vi "NIIE_lv_icon.vi"(10 "Color Icon":T4={"image type"=0, "image depth"=8, "image"=[255, 255, 255, 255, 255, 255, 255, 255, 255, 255, 255, 255, 255, 255, 255, 255, 255, 255, 255, 255, 255, 255, 255, 255, 255, 255, 255, 255, 255, 255, 255, 255, 255, 0, 0, 0, 0, 0, 0, 0, 0, 0, 0, 0, 0, 0, 0, 0, 0, 0, 0, 0, 0, 0, 0, 0, 0, 0, 0, 0, 0, 0, 0, 255, 255, 0, 0, 0, 0, 0, 0, 0, 0, 0, 0, 0, 0, 0, 0, 0, 0, 0, 0, 0, 0, 0, 0, 0, 0, 0, 0, 0, 0, 0, 0, 255, 255, 0, 0, 255, 255, 255, 255, 255, 255, 255, 255, 255, 255, 255, 255, 255, 255, 255, 255, 255, 255, 255, 0, 0, 0, 0, 0, 0, 0, 0, 0, 255, 255, 0, 0, 255, 250, 250, 250, 250, 250, 250, 250, 250, 250, 250, 250, 250, 248, 250, 44, 250, 44, 255, 0, 0, 0, 0, 0, 0, 0, 0, 0, 255, 255, 0, 0, 255, 250, 255, 255, 255, 255, 255, 255, 255, 255, 255, 255, 255, 248, 250, 44, 250, 44, 255, 0, 0, 0, 0, 0, 0, 0, 0, 0, 255, 255, 0, 0, 255, 250, 255, 209, 197, 209, 255, 255, 255, 209, 197, 209, 255, 248, 252, 43, 252, 44, 255, 0, 0, 0, 0, 0, 0, 0, 0, 0, 255, 255, 0, 0, 255, 250, 255, 197, 255, 197, 255, 255, 255, 197, 255, 197, 255, 248, 44, 44, 44, 44, 255, 0, 0, 0, 0, 0, 0, 0, 0, 0, 255, 255, 0, 0, 255, 250, 209, 197, 255, 197, 209, 255, 209, 197, 255, 197, 209, 248, 43, 252, 43, 44, 255, 0, 0, 0, 0, 0, 0, 0, 0, 0, 255, 255, 0, 0, 255, 250, 197, 209, 255, 209, 197, 255, 197, 209, 255, 209, 197, 248, 252, 8, 252, 44, 255, 0, 0, 0, 0, 0, 0, 0, 0, 0, 255, 255, 0, 0, 255, 250, 197, 255, 255, 255, 197, 255, 197, 255, 255, 255, 197, 248, 252, 8, 252, 44, 255, 0, 0, 0, 0, 0, 0, 0, 0, 0, 255, 255, 0, 0, 255, 250, 255, 255, 255, 255, 209, 197, 209, 255, 255, 255, 255, 248, 43, 252, 43, 44, 255, 0, 0, 0, 0, 0, 0, 0, 0, 0, 255, 255, 0, 0, 255, 250, 255, 255, 255, 255, 255, 255, 255, 255, 255, 255, 255, 248, 44, 44, 44, 44, 255, 0, 0, 0, 0, 0, 0, 0, 0, 0, 255, 255, 0, 0, 255, 248, 248, 248, 248, 248, 248, 248, 248, 248, 248, 248, 248, 248, 44, 44, 131, 131, 255, 0, 0, 0, 0, 0, 0, 0, 0, 0, 255, 255, 0, 0, 255, 44, 44, 44, 44, 44, 44, 44, 44, 44, 44, 44, 44, 44, 44, 44, 131, 5, 131, 131, 0, 0, 0, 0, 0, 0, 0, 0, 255, 255, 0, 0, 255, 44, 252, 44, 44, 44, 44, 44, 252, 44, 44, 44, 44, 35, 35, 35, 131, 5, 5, 5, 131, 131, 0, 0, 0, 0, 0, 0, 255, 255, 0, 0, 255, 252, 213, 252, 44, 44, 44, 252, 35, 252, 44, 35, 35, 44, 44, 44, 131, 5, 5, 255, 5, 5, 131, 131, 0, 0, 0, 0, 255, 255, 0, 0, 255, 44, 212, 44, 44, 44, 44, 35, 44, 44, 35, 44, 44, 44, 44, 44, 131, 5, 255, 255, 255, 5, 5, 5, 131, 35, 35, 0, 255, 255, 0, 0, 255, 255, 213, 255, 255, 255, 35, 255, 255, 35, 255, 255, 255, 255, 255, 255, 131, 5, 5, 255, 5, 5, 131, 131, 0, 0, 0, 0, 255, 255, 0, 0, 0, 0, 212, 0, 0, 0, 35, 0, 0, 35, 0, 0, 213, 212, 212, 213, 131, 5, 5, 5, 131, 131, 0, 0, 0, 0, 0, 0, 255, 255, 0, 0, 0, 0, 0, 213, 0, 0, 0, 35, 35, 0, 0, 212, 0, 0, 0, 0, 131, 5, 131, 131, 0, 0, 0, 0, 0, 0, 0, 0, 255, 255, 0, 0, 0, 0, 0, 0, 212, 212, 0, 0, 0, 0, 213, 0, 0, 0, 0, 0, 131, 131, 0, 0, 0, 0, 0, 0, 0, 0, 0, 0, 255, 255, 0, 0, 0, 0, 0, 0, 0, 0, 213, 212, 213, 212, 0, 0, 0, 0, 0, 0, 0, 0, 0, 0, 0, 0, 255, 255, 0, 0, 0, 0, 255, 255, 0, 0, 0, 0, 0, 0, 0, 0, 0, 0, 0, 0, 0, 0, 0, 0, 0, 0, 0, 0, 0, 0, 0, 255, 0, 0, 255, 0, 0, 0, 255, 255, 0, 0, 0, 0, 0, 0, 0, 0, 0, 0, 0, 0, 0, 0, 0, 0, 0, 0, 0, 0, 0, 0, 0, 0, 0, 0, 255, 0, 0, 0, 255, 255, 0, 0, 0, 0, 0, 0, 0, 0, 0, 0, 0, 0, 0, 0, 0, 0, 0, 0, 0, 0, 0, 0, 0, 0, 255, 255, 0, 0, 0, 0, 255, 255, 0, 0, 0, 0, 0, 0, 0, 0, 0, 0, 0, 0, 0, 0, 0, 0, 0, 0, 0, 0, 0, 0, 0, 0, 0, 0, 255, 0, 0, 0, 255, 255, 0, 0, 0, 0, 0, 0, 0, 0, 0, 0, 0, 0, 0, 0, 0, 0, 0, 0, 0, 0, 0, 0, 0, 255, 0, 0, 255, 0, 0, 0, 255, 255, 0, 0, 0, 0, 0, 0, 0, 0, 0, 0, 0, 0, 0, 0, 0, 0, 0, 0, 0, 0, 0, 0, 0, 0, 255, 255, 0, 0, 0, 0, 255, 255, 0, 0, 0, 0, 0, 0, 0, 0, 0, 0, 0, 0, 0, 0, 0, 0, 0, 0, 0, 0, 0, 0, 0, 0, 0, 0, 0, 0, 0, 0, 255, 255, 0, 0, 0, 0, 0, 0, 0, 0, 0, 0, 0, 0, 0, 0, 0, 0, 0, 0, 0, 0, 0, 0, 0, 0, 0, 0, 0, 0, 0, 0, 255, 255, 255, 255, 255, 255, 255, 255, 255, 255, 255, 255, 255, 255, 255, 255, 255, 255, 255, 255, 255, 255, 255, 255, 255, 255, 255, 255, 255, 255, 255, 255, 255], "mask"=[], "colors"=[16777215, 16777164, 16777113, 16777062, 16777011, 16776960, 16764159, 16764108, 16764057, 16764006, 16763955, 16763904, 16751103, 16751052, 16751001, 16750950, 16750899, 16750848, 16738047, 16737996, 16737945, 16737894, 16737843, 16737792, 16724991, 16724940, 16724889, 16724838, 16724787, 16724736, 16711935, 16711884, 16711833, 16711782, 16711731, 16711680, 13434879, 13434828, 13434777, 13434726, 13434675, 13434624, 13421823, 13421772, 13421721, 13421670, 13421619, 13421568, 13408767, 13408716, 13408665, 13408614, 13408563, 13408512, 13395711, 13395660, 13395609, 13395558, 13395507, 13395456, 13382655, 13382604, 13382553, 13382502, 13382451, 13382400, 13369599, 13369548, 13369497, 13369446, 13369395, 13369344, 10092543, 10092492, 10092441, 10092390, 10092339, 10092288, 10079487, 10079436, 10079385, 10079334, 10079283, 10079232, 10066431, 10066380, 10066329, 10066278, 10066227, 10066176, 10053375, 10053324, 10053273, 10053222, 10053171, 10053120, 10040319, 10040268, 10040217, 10040166, 10040115, 10040064, 10027263, 10027212, 10027161, 10027110, 10027059, 10027008, 6750207, 6750156, 6750105, 6750054, 6750003, 6749952, 6737151, 6737100, 6737049, 6736998, 6736947, 6736896, 6724095, 6724044, 6723993, 6723942, 6723891, 6723840, 6711039, 6710988, 6710937, 6710886, 6710835, 6710784, 6697983, 6697932, 6697881, 6697830, 6697779, 6697728, 6684927, 6684876, 6684825, 6684774, 6684723, 6684672, 3407871, 3407820, 3407769, 3407718, 3407667, 3407616, 3394815, 3394764, 3394713, 3394662, 3394611, 3394560, 3381759, 3381708, 3381657, 3381606, 3381555, 3381504, 3368703, 3368652, 3368601, 3368550, 3368499, 3368448, 3355647, 3355596, 3355545, 3355494, 3355443, 3355392, 3342591, 3342540, 3342489, 3342438, 3342387, 3342336, 65535, 65484, 65433, 65382, 65331, 65280, 52479, 52428, 52377, 52326, 52275, 52224, 39423, 39372, 39321, 39270, 39219, 39168, 26367, 26316, 26265, 26214, 26163, 26112, 13311, 13260, 13209, 13158, 13107, 13056, 255, 204, 153, 102, 51, 15597568, 14483456, 12255232, 11141120, 8912896, 7798784, 5570560, 4456448, 2228224, 1114112, 60928, 56576, 47872, 43520, 34816, 30464, 21760, 17408, 8704, 4352, 238, 221, 187, 170, 136, 119, 85, 68, 34, 17, 15658734, 14540253, 12303291, 11184810, 8947848, 7829367, 5592405, 4473924, 2236962, 1118481, 0], "Rectangle"={"left"=0, "top"=0, "right"=32, "bottom"=32}}, 11 "BW Icon":T4={"image type"=0, "image depth"=1, "image"=[255, 255, 255, 255, 128, 0, 0, 1, 128, 0, 0, 1, 159, 255, 252, 1, 144, 0, 84, 1, 151, 255, 84, 1, 150, 251, 84, 1, 149, 117, 4, 1, 149, 117, 36, 1, 147, 174, 84, 1, 147, 174, 84, 1, 151, 223, 36, 1, 151, 255, 4, 1, 144, 0, 28, 1, 144, 0, 22, 1, 148, 16, 241, 129, 158, 59, 18, 97, 148, 36, 23, 29, 159, 255, 242, 97, 132, 73, 241, 129, 130, 50, 22, 1, 129, 132, 24, 1, 128, 120, 0, 97, 128, 0, 0, 145, 128, 0, 0, 17, 128, 0, 0, 97, 128, 0, 0, 17, 128, 0, 0, 145, 128, 0, 0, 97, 128, 0, 0, 1, 128, 0, 0, 1, 255, 255, 255, 255], "mask"=[], "colors"=[16777215, 0], "Rectangle"={"left"=0, "top"=0, "right"=32, "bottom"=32}}) -> (0 "Error Code Out":i32=43, 2 "Color Icon Out":T4={"image type"=0, "image depth"=24, "image"=array[3072 elements], "mask"=[0, 0, 0, 0, 0, 0, 0, 0, 0, 0, 0, 0, 0, 0, 0, 0, 0, 0, 0, 0, 0, 0, 0, 0, 0, 0, 0, 0, 0, 0, 0, 0, 0, 0, 0, 0, 0, 0, 0, 0, 0, 0, 0, 0, 0, 0, 0, 0, 0, 0, 0, 0, 0, 0, 0, 0, 0, 0, 0, 0, 0, 0, 0, 0, 0, 0, 0, 0, 0, 0, 0, 0, 0, 0, 0, 0, 0, 0, 0, 0, 0, 0, 0, 0, 0, 0, 0, 0, 0, 0, 0, 0, 0, 0, 0, 0, 0, 0, 0, 0, 0, 0, 0, 0, 0, 0, 0, 0, 0, 0, 0, 0, 0, 0, 0, 0, 0, 0, 0, 0, 0, 0, 0, 0, 0, 0, 0, 0], "colors"=[], "Rectangle"={"left"=0, "top"=0, "right"=32, "bottom"=32}}, 3 "BW Icon Out":T4={"image type"=0, "image depth"=1, "image"=[0, 0, 0, 0, 0, 0, 0, 0, 0, 0, 0, 0, 0, 0, 0, 0, 0, 0, 0, 0, 0, 0, 0, 0, 0, 0, 0, 0, 0, 0, 0, 0, 0, 0, 0, 0, 0, 0, 0, 0, 0, 0, 0, 0, 0, 0, 0, 0, 0, 0, 0, 0, 0, 0, 0, 0, 0, 0, 0, 0, 0, 0, 0, 0, 0, 0, 0, 0, 0, 0, 0, 0, 0, 0, 0, 0, 0, 0, 0, 0, 0, 0, 0, 0, 0, 0, 0, 0, 0, 0, 0, 0, 0, 0, 0, 0, 0, 0, 0, 0, 0, 0, 0, 0, 0, 0, 0, 0, 0, 0, 0, 0, 0, 0, 0, 0, 0, 0, 0, 0, 0, 0, 0, 0, 0, 0, 0, 0], "mask"=[], "colors"=[16777215, 0], "Rectangle"={"left"=0, "top"=0, "right"=32, "bottom"=32}})   [LabVIEW 2021, in "lv_icon.lvlib"]
doc: "<p>Display this dialog box in one of the following ways:</p>\n\n<ul>\n<li>Double-click the <a href=\"nihelplauncher://docs/csh?context=lvcore_lvconcepts_using_icons\">icon</a> in the upper right corner of the front panel window, block diagram window, or <a href=\"nihelplauncher://docs/csh?context=lvcore_lvconcepts_custom_cont_ind_type\">Control Editor</a> window.</li>\n<li>Right-click the icon in the upper right corner of the front panel window, block diagram window, or <strong>Control Editor</strong> window and select <strong>Edit Icon</strong> from the shortcut menu.</li>\n<li>Select <strong>File<span class=\"U+187\">>></span>VI Properties</strong> or <strong>File<span class=\"U+187\">>></span>Control Properties</strong> to display the <a href=\"nihelplauncher://docs/csh?context=lvcore_lvdialog_vi_properties_dialog_box\">VI Properties</a> dialog box or <strong>Control Properties</strong> dialog box, respectively. Then select <strong>General</strong> from the <strong>Category</strong> pull-down menu and click the <strong>Edit Icon</strong> button.</li>\n<li>Right-click a project library, statechart, class, or XControl item in the <a href=\"nihelplauncher://docs/csh?context=lvcore_lvconcepts_using_labview_projects\">Project Explorer</a> window and select <strong> Properties</strong> from the shortcut menu to display the corresponding <strong>Properties</strong> dialog box. Then click the <strong>Edit</strong> button on the <strong>General Settings</strong> page.</li>\n</ul>\n\n<p>Use this dialog box to <a href=\"nihelplauncher://docs/csh?context=lvcore_lvhowto_creating_icons\">create and edit icons</a>.</p>"
uses:
  vi.lib/LabVIEW Icon API/lv_icon/lv_icon.lvlib
  MB CORE/TypeDefs/Cluster_BodyText.ctl
  vi.lib/LabVIEW Icon API/lv_icon/Controls/Font.ctl
  vi.lib/LabVIEW Icon API/lv_icon/Controls/Alignment.ctl
  MB CORE/TypeDefs/Cluster_Layer Data.ctl
  NIIconEditor/Controls/LayerList.ctl
  NIIconEditor/Controls/NewLayer.ctl
  NIIconEditor/Controls/DeleteLayer.ctl
  NIIconEditor/Controls/Arrow Up.ctl
  NIIconEditor/Controls/Arrow Down.ctl
  NIIconEditor/Controls/Framework Templates.ctl
  vi.lib/LabVIEW Icon API/lv_icon/Controls/Graphic.ctl
  NIIconEditor/Controls/ColorChange.ctl
  vi.lib/LabVIEW Icon API/lv_icon/Controls/IEColor.ctl
  NIIconEditor/Controls/Rotate.ctl
  NIIconEditor/Controls/Flip.ctl
  MB CORE/TypeDefs/Cluster_Button Draw Tools.ctl
  MB CORE/TypeDefs/Bool_Draw Tool.ctl
  MB CORE/TypeDefs/Bool_Line Tool.ctl
  MB CORE/TypeDefs/Bool_ColorExtractor Tool.ctl
  MB CORE/TypeDefs/Bool_Fill Tool.ctl
  MB CORE/TypeDefs/Bool_IERect Tool.ctl
  MB CORE/TypeDefs/Bool_FRect Tool.ctl
  MB CORE/TypeDefs/Bool_Circle Tool.ctl
  MB CORE/TypeDefs/Bool_FillCircle Tool.ctl
  MB CORE/TypeDefs/Bool_Eraser Tool.ctl
  MB CORE/TypeDefs/Bool_Text Tool.ctl
  MB CORE/TypeDefs/Bool_Selection Tool.ctl
  MB CORE/TypeDefs/Bool_Move Tool.ctl
  MB CORE/TypeDefs/String_TextMarker Tool.ctl
  <vilib>/picture/picture.llb/imagedata.ctl
  MB CORE/TypeDefs/Cluster_Path&Icon.ctl
  NIIconEditor/Controls/Refresh.ctl
  <vilib>/Utility/miscctls.llb/LVKeyNavTypeDef.ctl
  NIIconEditor/Controls/References Cluster.ctl
  <vilib>/Utility/miscctls.llb/LVPoint32TypeDef.ctl
  <vilib>/Utility/miscctls.llb/LVPositionTypeDef.ctl
  vi.lib/LabVIEW Icon API/lv_icon/Controls/Pathes.ctl
  NIIconEditor/Class/Ants/Ants.lvclass
  NIIconEditor/Class/FakedArray/FakedArray.lvclass
  vi.lib/LabVIEW Icon API/lv_icon/Classes/Icon/Icon.lvclass
  NIIconEditor/Class/Icon Library/Glyph.lvclass
  <resource>/dialog/lvconfig.llb/LV Config Read String.vi
  <resource>/dialog/lvconfig.llb/LV Config Write String.vi
panel:
  out "LabVIEW Icon out":string
  in  "LabVIEW Icon in":string
  out "Terminals":picture
  out "Preview2":picture
  in  "?":cluster{T1[], i32, bool}
  out "TextMarker":T2="^"
  in  "Help":bool
  in  "Cancel":bool
  in  "OK":bool
  out "XYZ":string="X: 14\nY: 31\nZ: 1"
  out "RGB":string="R: 0\nG: 0\nB: 0"
  out "Icon":picture
  out "Clipboard":picture
  in  "?":T3[](array[typedef])
  in  "Tab Control":T5(tab)
  in  "refreshTemplates":T6
  out "templates path str":string
  in  "Templates":string(tree)="<All>"
  in  "Filter templates by keyword":string
  in  "Framework Templates":T7={"Scrollbar"=0, "Path & Icon 1"={"Rectangle"={"left"=0, "top"=0, "right"=32, "bottom"=32}, "Path"=path "C:/Users/tsandris/Documents/LabVIEW Data/Icon Templates/VI/Frameworks/_blank.png", "Image"=bytes[3230], "Filter"="VI\\Frameworks", "FileName"="_blank"}, "Path & Icon 2"={"Rectangle"={"left"=0, "top"=0, "right"=32, "bottom"=32}, "Path"=path "C:/Users/tsandris/Documents/LabVIEW Data/Icon Templates/Library/Frameworks/_blank.png", "Image"=bytes[3230], "Filter"="Library\\Frameworks", "FileName"="_blank"}, "Path & Icon 3"={"Rectangle"={"left"=0, "top"=0, "right"=0, "bottom"=0}, "Path"=path "", "Image"=bytes[0], "Filter"="", "FileName"=""}, "Path & Icon 4"={"Rectangle"={"left"=0, "top"=0, "right"=0, "bottom"=0}, "Path"=path "", "Image"=bytes[0], "Filter"="", "FileName"=""}, "Path & Icon 5"={"Rectangle"={"left"=0, "top"=0, "right"=0, "bottom"=0}, "Path"=path "", "Image"=bytes[0], "Filter"="", "FileName"=""}, "Path & Icon 6"={"Rectangle"={"left"=0, "top"=0, "right"=0, "bottom"=0}, "Path"=path "", "Image"=bytes[0], "Filter"="", "FileName"=""}, "Path & Icon 7"={"Rectangle"={"left"=0, "top"=0, "right"=0, "bottom"=0}, "Path"=path "", "Image"=bytes[0], "Filter"="", "FileName"=""}, "Path & Icon 8"={"Rectangle"={"left"=0, "top"=0, "right"=0, "bottom"=0}, "Path"=path "", "Image"=bytes[0], "Filter"="", "FileName"=""}, "Path & Icon 9"={"Rectangle"={"left"=0, "top"=0, "right"=0, "bottom"=0}, "Path"=path "", "Image"=bytes[0], "Filter"="", "FileName"=""}, "Path & Icon 10"={"Rectangle"={"left"=0, "top"=0, "right"=0, "bottom"=0}, "Path"=path "", "Image"=bytes[0], "Filter"="", "FileName"=""}, "Path & Icon 11"={"Rectangle"={"left"=0, "top"=0, "right"=0, "bottom"=0}, "Path"=path "", "Image"=bytes[0], "Filter"="", "FileName"=""}, "Path & Icon 12"={"Rectangle"={"left"=0, "top"=0, "right"=0, "bottom"=0}, "Path"=path "", "Image"=bytes[0], "Filter"="", "FileName"=""}, "Path & Icon 13"={"Rectangle"={"left"=0, "top"=0, "right"=0, "bottom"=0}, "Path"=path "", "Image"=bytes[0], "Filter"="", "FileName"=""}, "Path & Icon 14"={"Rectangle"={"left"=0, "top"=0, "right"=0, "bottom"=0}, "Path"=path "", "Image"=bytes[0], "Filter"="", "FileName"=""}, "Path & Icon 15"={"Rectangle"={"left"=0, "top"=0, "right"=0, "bottom"=0}, "Path"=path "", "Image"=bytes[0], "Filter"="", "FileName"=""}, "Path & Icon 16"={"Rectangle"={"left"=0, "top"=0, "right"=0, "bottom"=0}, "Path"=path "", "Image"=bytes[0], "Filter"="", "FileName"=""}, "Path & Icon 17"={"Rectangle"={"left"=0, "top"=0, "right"=0, "bottom"=0}, "Path"=path "", "Image"=bytes[0], "Filter"="", "FileName"=""}, "Path & Icon 18"={"Rectangle"={"left"=0, "top"=0, "right"=0, "bottom"=0}, "Path"=path "", "Image"=bytes[0], "Filter"="", "FileName"=""}, "Path & Icon 19"={"Rectangle"={"left"=0, "top"=0, "right"=0, "bottom"=0}, "Path"=path "", "Image"=bytes[0], "Filter"="", "FileName"=""}, "Path & Icon 20"={"Rectangle"={"left"=0, "top"=0, "right"=0, "bottom"=0}, "Path"=path "", "Image"=bytes[0], "Filter"="", "FileName"=""}, "Path & Icon 21"={"Rectangle"={"left"=0, "top"=0, "right"=0, "bottom"=0}, "Path"=path "", "Image"=bytes[0], "Filter"="", "FileName"=""}, "Path & Icon 22"={"Rectangle"={"left"=0, "top"=0, "right"=0, "bottom"=0}, "Path"=path "", "Image"=bytes[0], "Filter"="", "FileName"=""}, "Path & Icon 23"={"Rectangle"={"left"=0, "top"=0, "right"=0, "bottom"=0}, "Path"=path "", "Image"=bytes[0], "Filter"="", "FileName"=""}, "Path & Icon 24"={"Rectangle"={"left"=0, "top"=0, "right"=0, "bottom"=0}, "Path"=path "", "Image"=bytes[0], "Filter"="", "FileName"=""}, "Path & Icon 25"={"Rectangle"={"left"=0, "top"=0, "right"=0, "bottom"=0}, "Path"=path "", "Image"=bytes[0], "Filter"="", "FileName"=""}, "Path & Icon 26"={"Rectangle"={"left"=0, "top"=0, "right"=0, "bottom"=0}, "Path"=path "", "Image"=bytes[0], "Filter"="", "FileName"=""}, "Path & Icon 27"={"Rectangle"={"left"=0, "top"=0, "right"=0, "bottom"=0}, "Path"=path "", "Image"=bytes[0], "Filter"="", "FileName"=""}, "Path & Icon 28"={"Rectangle"={"left"=0, "top"=0, "right"=0, "bottom"=0}, "Path"=path "", "Image"=bytes[0], "Filter"="", "FileName"=""}, "Path & Icon 29"={"Rectangle"={"left"=0, "top"=0, "right"=0, "bottom"=0}, "Path"=path "", "Image"=bytes[0], "Filter"="", "FileName"=""}, "Path & Icon 30"={"Rectangle"={"left"=0, "top"=0, "right"=0, "bottom"=0}, "Path"=path "", "Image"=bytes[0], "Filter"="", "FileName"=""}}
  in  "Body Text":T8={"Line 1 text"="", "Line 2 text"="", "Line 3 text"="", "Line 4 text"="", "Line 1 color"=0, "Line 2 color"=0, "Line 3 color"=0, "Line 4 color"=0, "Body Text Spec"={"Font"="", "Alignment"=1, "Size"=9}, "Center text vertically"=TRUE, "Capitalize Text"=TRUE} {"Body Text Spec"."Alignment" items=["left", "center", "right"]}
  in  "Filter glyphs by keyword":string
  in  "Glyphs":string(tree)="<All>"
  out "glyph path str":string
  out "Glyphs []":T1[][](array[typedef])
  in  "refreshGlyphs":T6
  in  "Add Layer":T11
  in  "Remove Layer":T12
  in  "Move Down":T13
  in  "Move Up":T14
  in  "Icon Template":T15={"LayerIcon"=bytes[0], "LayerName"="", "Opacity"=100, "Visibility?"=TRUE} {"Opacity" scale=0.0..100.0}
  in  "Icon Text":T15={"LayerIcon"=bytes[0], "LayerName"="Icon Text", "Opacity"=100, "Visibility?"=TRUE} {"Opacity" scale=0.0..100.0}
  in  "User Layers":T16={"Scrollbar"=0, "Layer 1"={"LayerIcon"=bytes[3230], "LayerName"="VI Icon", "Opacity"=100, "Visibility?"=TRUE}, "Layer 2"={"LayerIcon"=bytes[3230], "LayerName"="", "Opacity"=100, "Visibility?"=TRUE}, "Layer 3"={"LayerIcon"=bytes[3230], "LayerName"="", "Opacity"=100, "Visibility?"=TRUE}, "Layer 4"={"LayerIcon"=bytes[3230], "LayerName"="", "Opacity"=100, "Visibility?"=TRUE}} {"Layer 4"."Opacity" scale=0.0..100.0; "Layer 3"."Opacity" scale=0.0..100.0; "Layer 2"."Opacity" scale=0.0..100.0; "Layer 1"."Opacity" scale=0.0..100.0}
  out "Preview":picture
  in  "Horizontal Flip":T17
  in  "Clockwise Rotate":T18
  in  "Swap":T19
  in  "Line Color":T20
  in  "Fill Color":T20=16777215
  in  "Tools":T21=enum."Rectangle"
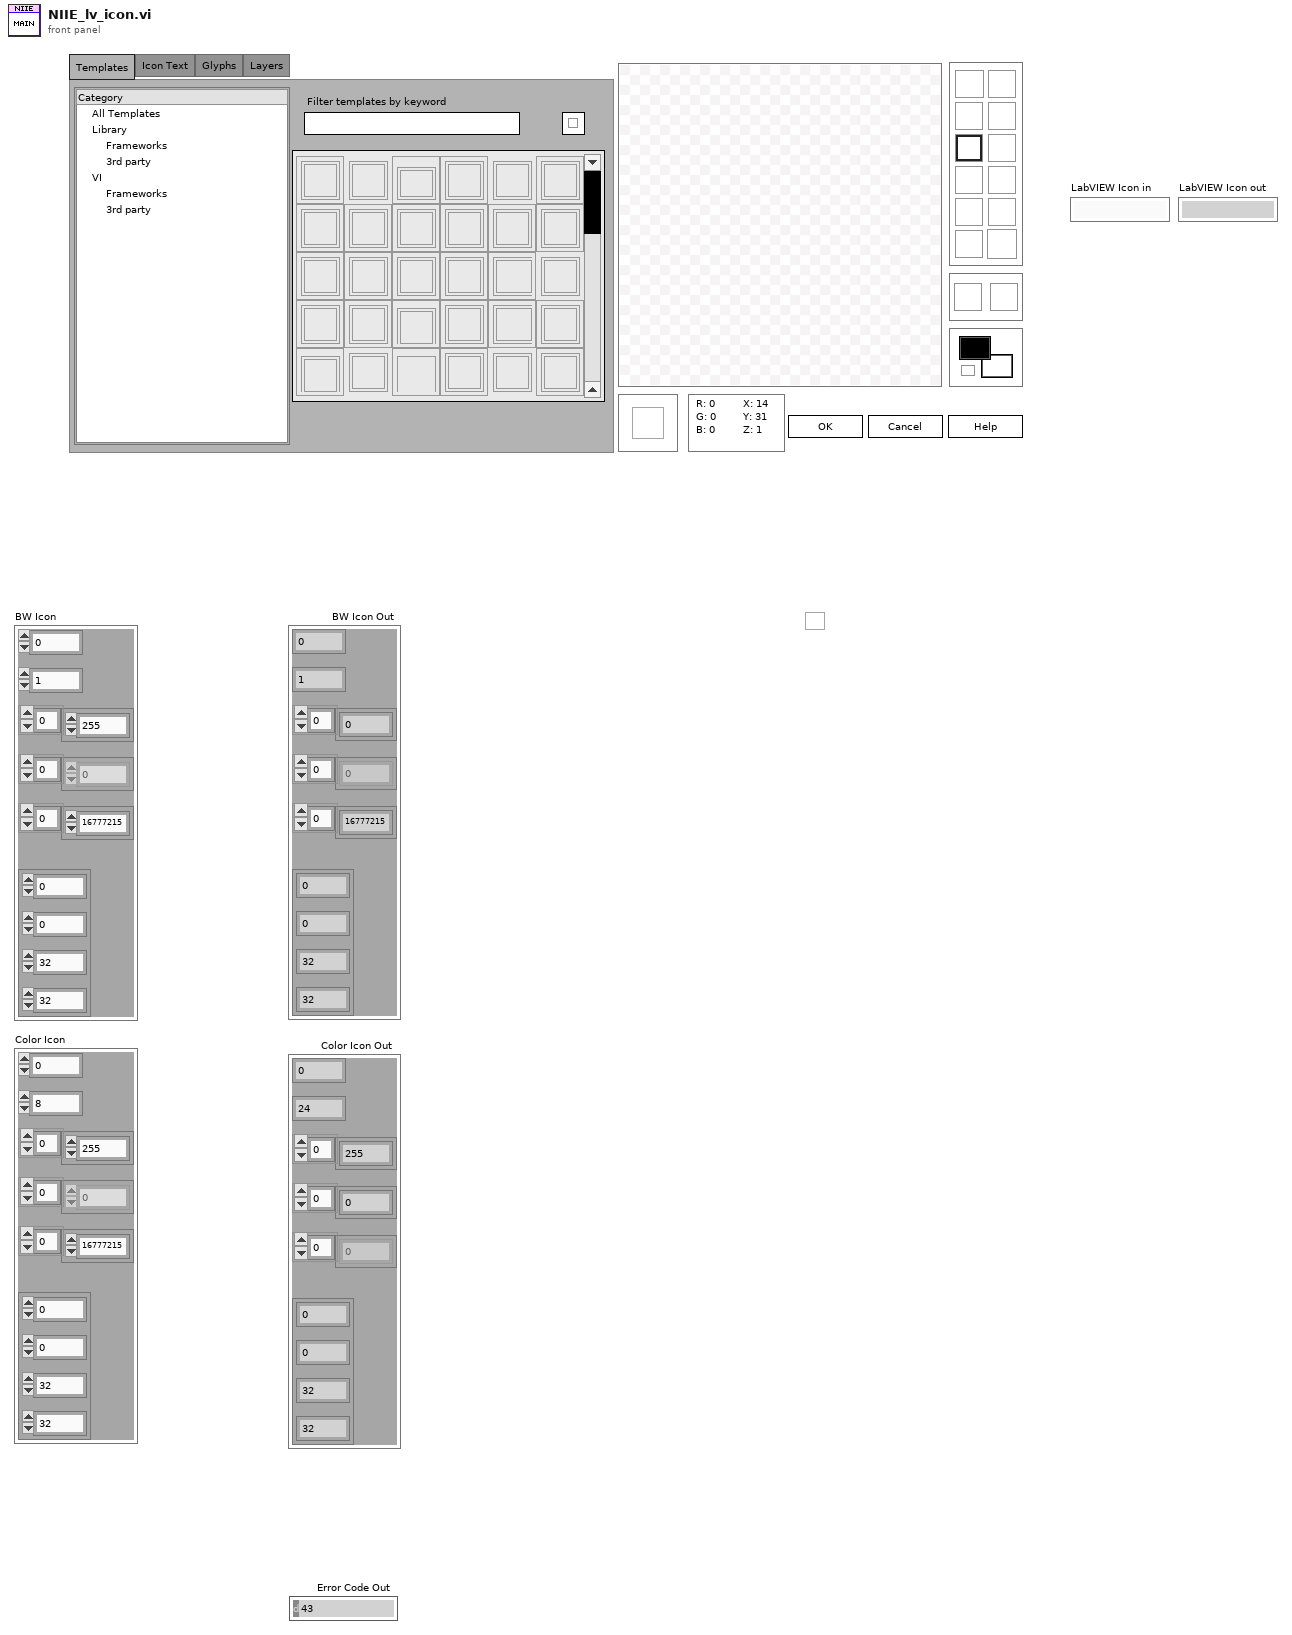
[diagram p1: front panel]
types:
  T1 = typedef "Graphic.ctl" = cluster{"Rectangle":cluster{"left":i16, "top":i16, "right":i16, "bottom":i16}, "Path":path, "Image":picture, "Filter":string, "FileName":string}
  T2 = typedef "String_TextMarker Tool.ctl" = string
  T3 = typedef "Cluster_Path&Icon.ctl" = cluster{"Rectangle":cluster{"left":i16, "top":i16, "right":i16, "bottom":i16}, "Path":path, "Image":picture, "Filter":string, "FileName":string}
  T4 = typedef "imagedata.ctl" = cluster{"image type":i32, "image depth":i32, "image":u8[], "mask":u8[], "colors":u32[], "Rectangle":cluster{"left":i16, "top":i16, "right":i16, "bottom":i16}}
  T5 = enum32{"Templates", "Icon Text", "Glyphs", "Layers"}
  T6 = typedef "Refresh.ctl" = bool
  T7 = typedef "Framework Templates.ctl" = cluster{"Scrollbar":i32, "Path & Icon 1":T1, "Path & Icon 2":T1, "Path & Icon 3":T1, "Path & Icon 4":T1, "Path & Icon 5":T1, "Path & Icon 6":T1, "Path & Icon 7":T1, "Path & Icon 8":T1, "Path & Icon 9":T1, "Path & Icon 10":T1, "Path & Icon 11":T1, "Path & Icon 12":T1, "Path & Icon 13":T1, "Path & Icon 14":T1, "Path & Icon 15":T1, "Path & Icon 16":T1, "Path & Icon 17":T1, "Path & Icon 18":T1, "Path & Icon 19":T1, "Path & Icon 20":T1, "Path & Icon 21":T1, "Path & Icon 22":T1, "Path & Icon 23":T1, "Path & Icon 24":T1, "Path & Icon 25":T1, "Path & Icon 26":T1, "Path & Icon 27":T1, "Path & Icon 28":T1, "Path & Icon 29":T1, "Path & Icon 30":T1}
  T8 = typedef "Cluster_BodyText.ctl" = cluster{"Line 1 text":string, "Line 2 text":string, "Line 3 text":string, "Line 4 text":string, "Line 1 color":u32, "Line 2 color":u32, "Line 3 color":u32, "Line 4 color":u32, "Body Text Spec":cluster{"Font":T9, "Alignment":T10, "Size":u8}, "Center text vertically":bool, "Capitalize Text":bool}
  T9 = typedef "Font.ctl" = string
  T10 = typedef "Alignment.ctl" = u16
  T11 = typedef "NewLayer.ctl" = bool
  T12 = typedef "DeleteLayer.ctl" = bool
  T13 = typedef "Arrow Down.ctl" = bool
  T14 = typedef "Arrow Up.ctl" = bool
  T15 = typedef "Cluster_Layer Data.ctl" = cluster{"LayerIcon":picture, "LayerName":string, "Opacity":u8, "Visibility?":bool}
  T16 = typedef "LayerList.ctl" = cluster{"Scrollbar":i32, "Layer 1":T15, "Layer 2":T15, "Layer 3":T15, "Layer 4":T15}
  T17 = typedef "Flip.ctl" = bool
  T18 = typedef "Rotate.ctl" = bool
  T19 = typedef "ColorChange.ctl" = bool
  T20 = typedef "IEColor.ctl" = u32
  T21 = typedef "Cluster_Button Draw Tools.ctl" = enum32{"Pencil", "Line", "Dropper", "Fill", "Rectangle", "Filled Rectangle", "Ellipse", "Filled Ellipse", "Eraser", "Text", "Select", "Move"}
  T22 = enum32{"Invalid", "Standard", "Closed", "Hidden", "Minimized", "Maximized"}
  T23 = typedef "References Cluster.ctl" = cluster{"Add Layer":refnum<vi>, "Remove Layer":refnum<vi>, "Line Text":refnum<vi>[], "Body Text Spec":refnum<vi>, "DNL_Font":refnum<vi>, "glyph path str":refnum<vi>, "templates path str":refnum<vi>, "Arrow Up":refnum<vi>, "Arrow Down":refnum<vi>, "IE VI Ref":refnum<vi>, "Glyphs tree":refnum<vi>, "Templates tree":refnum<vi>, "Layer Icon Text":refnum<vi>, "Layer Template":refnum<vi>, "Clipboard":refnum<vi>, "BW icon in":refnum<vi>, "Color icon in":refnum<vi>, "Layer Clust":refnum<vi>, "Body Text":refnum<vi>, "DNL_Framework Templates":refnum<vi>, "Search Templates":refnum<vi>, "TextMarker":refnum<vi>, "Tab Control":refnum<vi>, "Search Glyphs":refnum<vi>, "Line Color":refnum<vi>, "DNL_Glyphs []":refnum<vi>, "Fill Color":refnum<vi>, "Tools":refnum<vi>, "Glyphs tree":refnum<vi>, "Icon":refnum<vi>, "Preview":refnum<vi>, "Ants":refnum<vi>, "Terminals":refnum<vi>, "menu reference":refnum<k9>, "LayerNames":refnum<vi>[], "GlyphLoadAnimation":refnum<vi>, "TemplateLoadAnimation":refnum<vi>, "refreshGlyphs":refnum<vi>, "refreshTemplates":refnum<vi>}
  T24 = typedef "LVKeyNavTypeDef.ctl" = cluster{"Control":bool, "Shift":bool, "Key":string}
  T25 = cluster{"Left":i16, "Top":i16, "Right":i16, "Bottom":i16}
  T26 = typedef "LVAllMonitorsDisplayTypeDef.ctl" = cluster{"Bounds":cluster{"Left":i16, "Top":i16, "Right":i16, "Bottom":i16}, "Depth":i16}[]
  T27 = cluster{"Global stop?":refnum<user-event>, "Templates":refnum<user-event>, "Glyphs":refnum<user-event>}
  T28 = typedef "IE Data.ctl" = cluster{"Class":T29, "Ref":T23, "Support":T30}
  T29 = typedef "IE Classes.ctl" = cluster{"Ants":refnum<class "Ants.lvclass">, "Layer":refnum<class "FakedArray.lvclass">, "Templates":refnum<class "FakedArray.lvclass">, "Icon":refnum<class "Icon.lvclass">, "Glyph":refnum<class "Glyph.lvclass">, "Settings":refnum<class "Settings.lvclass">, "Tools":refnum<class "Tools Paint.lvclass">}
  T30 = typedef "SupportClass.ctl" = cluster{"AntsRect":cluster{"left":i16, "top":i16, "right":i16, "bottom":i16}, "Mouse Move Coords":T31, "Mouse Down Coords":T31, "Temp Coord":T31, "Action":T32, "Edge Color":T20, "Fill Color":T20, "Mouse Down?":bool, "Draft Mode?":bool, "Temp Icon":picture, "CTRL Pressed":bool, "Move Selection?":bool, "AntsRect Orig":cluster{"left":i16, "top":i16, "right":i16, "bottom":i16}, "Text":string, "TM Set?":bool, "Mouse inside icon?":bool, "Tool (old value)":u32, "Pencil Move Color":u32, "Swap Colors?":bool, "Shift pressed?":bool}
  T31 = typedef "LVPoint32TypeDef.ctl" = cluster{"Horizontal":i32, "Vertical":i32}
  T32 = typedef "ENUM_SupportClass_Action.ctl" = enum16{"Default", "Move Selection", "Glyph Library", "Tool"}
  T33 = typedef "LVPositionTypeDef.ctl" = cluster{"Left":i32, "Top":i32}
  T34 = typedef "Pathes.ctl" = enum16{"Root Path", "Icon Templates", "Icon Templates VI", "Icon Templates Lib", "Glyphs"}
  T35 = typedef "lveventtype.ctl" = enum32{"Null", "Timeout", "Annotation Menu Selection", "Annotation Menu Selection?", "App Instance Close", "App Instance Close?", "Autoscale Range Change", "Bookmark Info Change", "Cell Edit", "Cell Edit?", "Cursor Grab", "Cursor Grab?", "Cursor Menu Selection", "Cursor Menu Selection?", "Cursor Move", "Cursor Release", "Data Change", "Direction Change", "Display State Change", "Drag Ended", "Drag Enter", "Drag Leave", "Drag Over", "Drag Source Update", "Drag Starting", "Drag Starting?", "Drop", "Exec State Change", "Key Down", "Key Down?", "Key Repeat", "Key Repeat?", "Key Up", "Listbox Double Click", "Menu Activation?", "Menu Selection (App)", "Menu Selection? (App)", "Menu Selection (User)", "Mouse Down", "Mouse Down?", "Mouse Enter", "Mouse Leave", "Mouse Move", "Mouse Up", "Mouse Wheel", "NI Security User Change (App)", "Pane Size", "Panel Close", "Panel Close?", "Panel Resize", "Plot Attribute Change", "Scale Range Change", "Shortcut Menu Activation?", "Shortcut Menu Selection (App)", "Shortcut Menu Selection? (App)", "Shortcut Menu Selection (User)", "Tree Double Click", "Tree Drag", "Tree Drag?", "Tree Drop", "Tree Drop?", "Tree Item Close", "Tree Item Close?", "Tree Item Open", "Tree Item Open?", "User Event", "Value Change"}
  T36 = typedef "eventvkey.ctl" = enum16{"ASCII", "Enter", "Return", "Shift", "Ctrl", "Alt", "Cmd", "Opt", "Caps", "NumLock", "Clear", "Break", "Up", "Down", "Left", "Right", "Insert", "Delete", "Home", "End", "PageUp", "PageDown", "Escape", "Help", "Pause", "ScrollLock", "F1", "F2", "F3", "F4", "F5", "F6", "F7", "F8", "F9", "F10", "F11", "F12", "F13", "F14", "F15", "F16", "F17", "F18", "F19", "F20", "F21", "F22", "F23", "F24", "Play", "VolumeUp", "VolumeDown", "Mute", "Two Byte Char"}
  T37 = cluster{"Shift":bool, "Ctrl":bool, "Alt":bool, "Cmd":bool, "Opt":bool}
  T38 = typedef "LVRectTypeDef.ctl" = cluster{"Left":i16, "Top":i16, "Right":i16, "Bottom":i16}
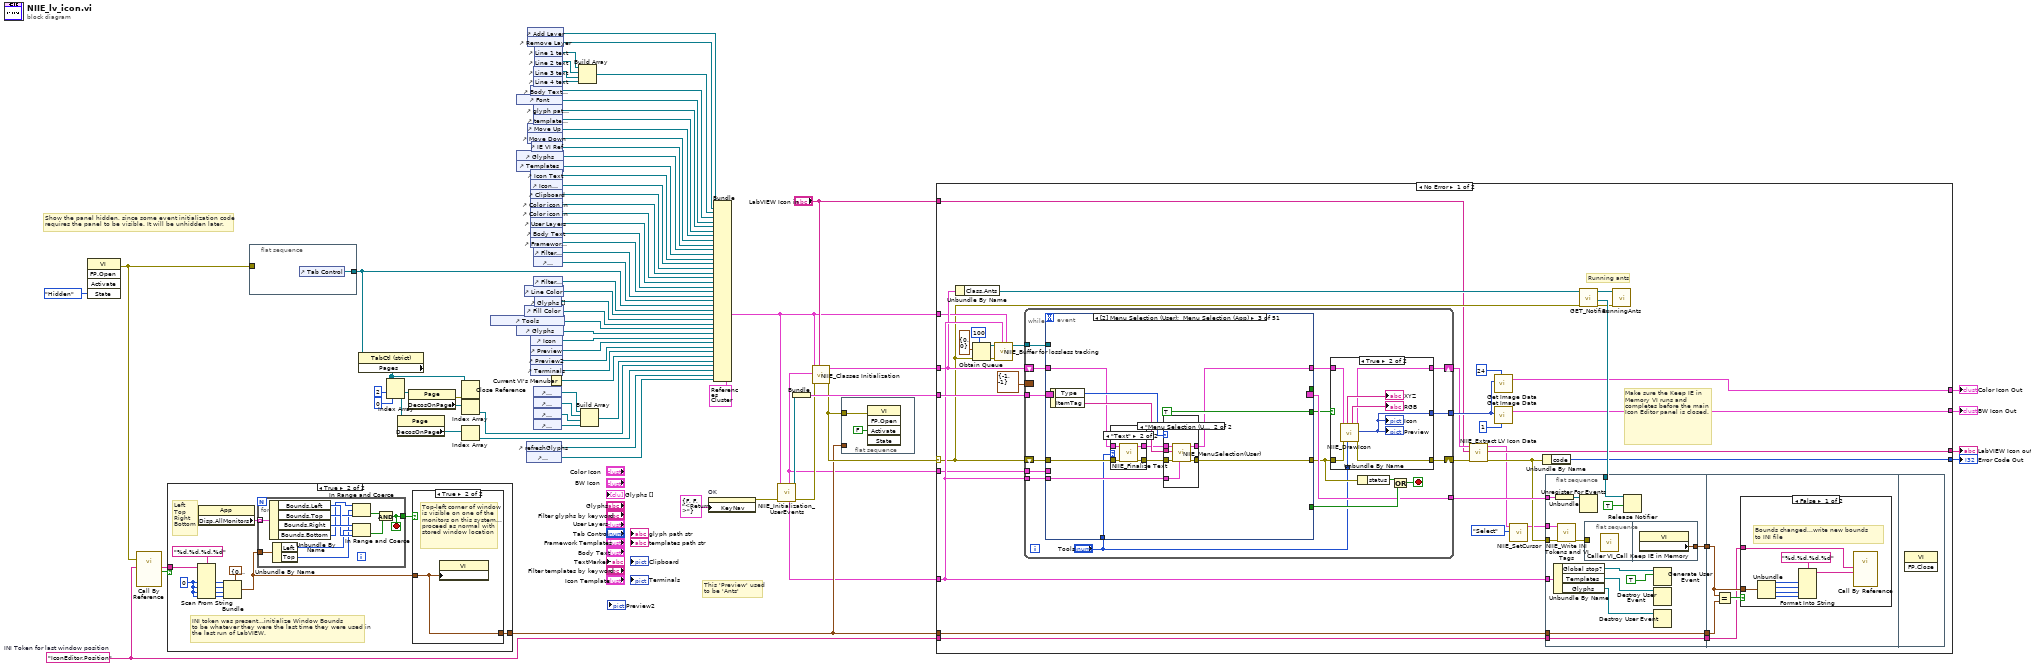
[diagram p0: block diagram]
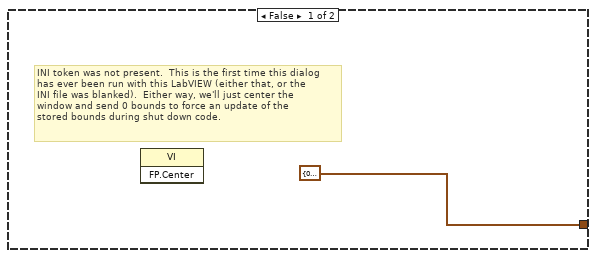
[diagram p2: hidden frame]
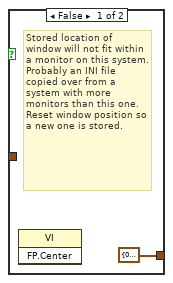
[diagram p3: hidden frame]
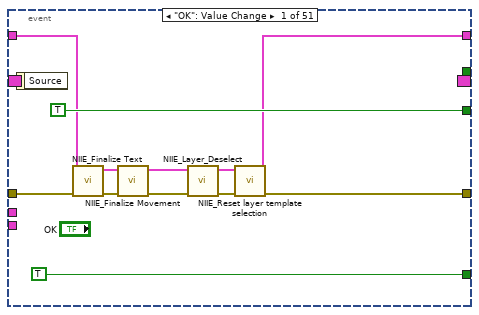
[diagram p4: hidden frame]
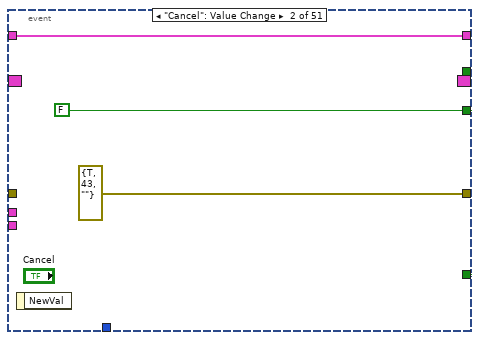
[diagram p5: hidden frame]
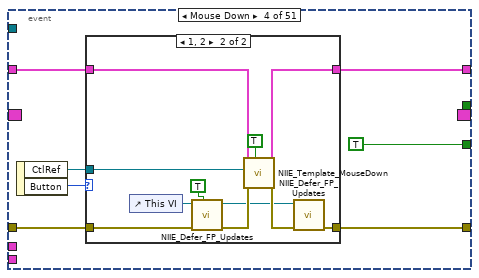
[diagram p8: hidden frame]
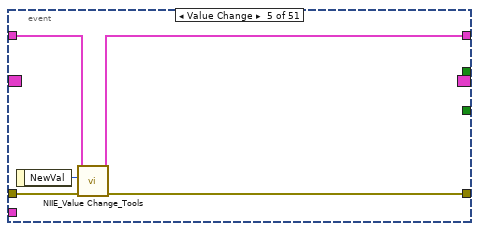
[diagram p10: hidden frame]
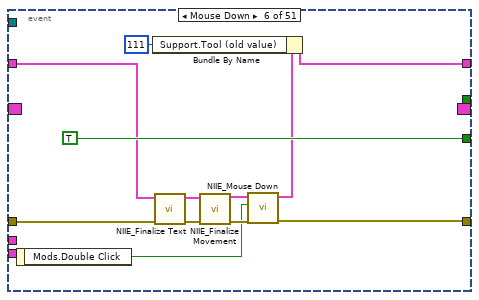
[diagram p11: hidden frame]
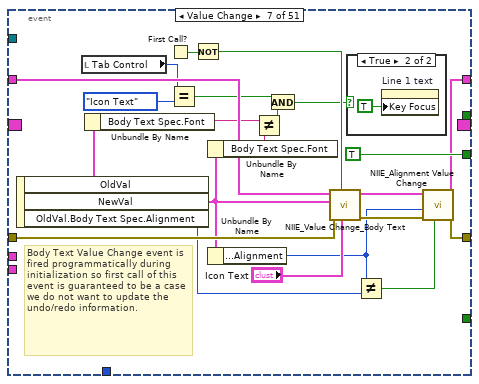
[diagram p12: hidden frame]
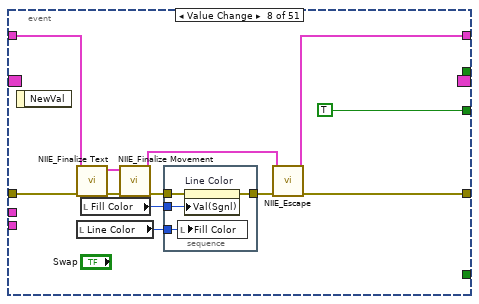
[diagram p14: hidden frame]
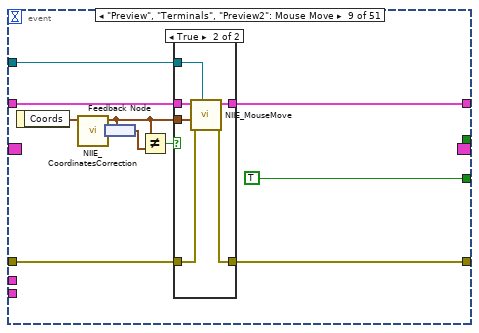
[diagram p15: hidden frame]
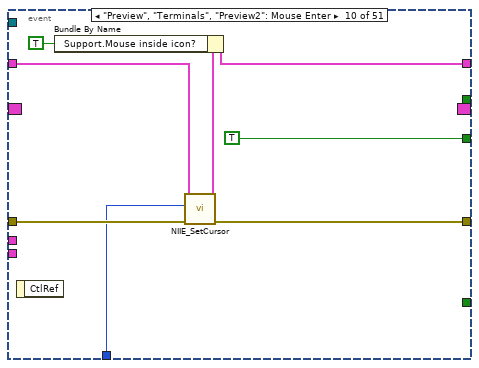
[diagram p17: hidden frame]
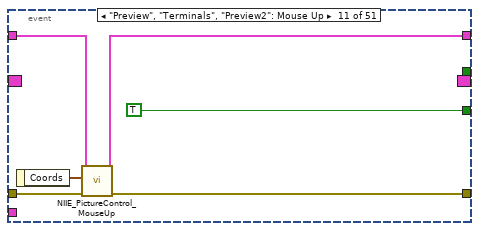
[diagram p18: hidden frame]
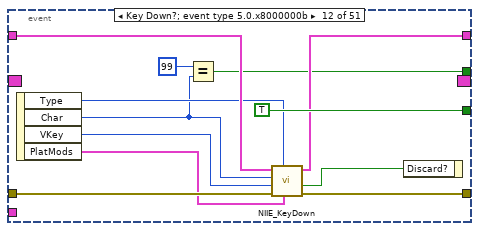
[diagram p19: hidden frame]
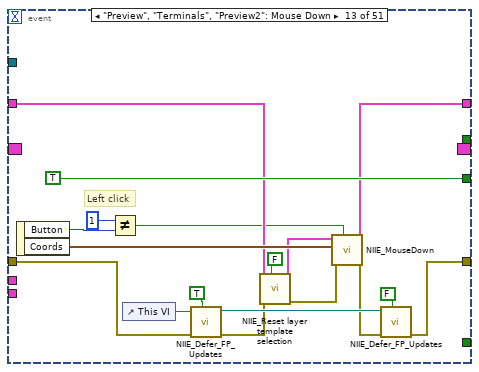
[diagram p20: hidden frame]
diagram:
  w2 = "IconEditor.Position"  # INI Token for last window position
  # "Show the panel hidden, since some event initialization code requires the panel to be visible. It will be unhidden later."
  # "This 'Preview' used\nto be 'Ants'"
  n1 = invoke class="VI" method="FP.Open"("State"=T22."Hidden") -> (error out=w4:errorcluster)  [unwired: 4 in, 4 out]
  n2 = call-by-ref "?"(error in=w4, "key"=w2) -> ("found?"=w5:bool, "value"=w6:string)  [unwired: 5 in, 3 out]
  n3 = case shown="True" w5 {
    tunnel: [T25 {"Left"=0, "Top"=0, "Right"=0, "Bottom"=0} ("Front Panel.PanelBounds") w78] -> w3
    tunnel: w6 -> [_ w89]
    frame False {
      # "INI token was not present.  This is the first time this dialog\nhas ever been run with this LabVIEW (either that, or the\nINI file was blanked).  Either way, we'll just center the\nwindow and send 0 bounds to force an update of the\nstored bounds during shut down code."
      n4 = invoke class="VI" method="FP.Center"() -> ()  [unwired: 3 in, 3 out]
    }
    frame True {
      w87 = i16 0 ("default value 1")
      # "Left\nTop\nRight\nBottom"
      # "INI token was present...initialize Window Bounds\nto be whatever they were the last time they were used in\nthe last run of LabVIEW."
      n5 = Scan From String(format string="%d,%d,%d,%d", input string=w89, default 1=w87, default 2=w87, default 3=w87, default 4=w87) -> (output 1=w86:i16, output 2=w85:i16, output 3=w84:i16, output 4=w83:i16)  [unwired: 2 in, 3 out]
      n6 = property class="App"() -> ("Disp.AllMonitors"=w81:T26)  [unwired: 2 in, 2 out]
      n7 = Bundle(cluster=T25 {"Left"=0, "Top"=0, "Right"=0, "Bottom"=0} ("Front Panel.PanelBounds"), "Left"=w86, "Top"=w85, "Right"=w84, "Bottom"=w83) -> (w80:T25)
      n8 = for {
        tunnel: w81 -> [w102] mode=indexing
        tunnel: w80 -> [w101]
        tunnel: [w92] -> w79
        stop <- w92 stop-if-true
        n9 = Unbundle By Name(w102) -> ("Bounds.Left"=w99:i16, "Bounds.Top"=w97:i16, "Bounds.Right"=w100:i16, "Bounds.Bottom"=w96:i16)
        n10 = Unbundle By Name(w101) -> ("Left"=w98:i16, "Top"=w95:i16)
        n11 = In Range and Coerce(upper limit=w96, x=w95, lower limit=w97) -> (In Range?=w94:bool)  [unwired: 1 out]
        n12 = In Range and Coerce(upper limit=w100, x=w98, lower limit=w99) -> (In Range?=w93:bool)  [unwired: 1 out]
        n13 = And(x=w94, y=w93) -> (x .and. y?=w92:bool)
      }
      n14 = case shown="True" w79 {
        tunnel: w80 -> [_ w91]
        tunnel: [T25 {"Left"=0, "Top"=0, "Right"=0, "Bottom"=0} ("Front Panel.PanelBounds") w91] -> w78
        frame False {
          # "Stored location of window will not fit within a monitor on this system.  Probably an INI file copied over from a system with more monitors than this one.  Reset window position so a new one is stored."
          n15 = invoke class="VI" method="FP.Center"() -> ()  [unwired: 3 in, 3 out]
        }
        frame True {
          # "Top-left corner of window is visible on one of the monitors on this system... proceed as normal with stored window location"
          n16 = property class="VI"("Front Panel.WinBounds"=w91) -> ()  [unwired: 2 in, 2 out]
        }
      }
    }
  }
  n17 = flat-sequence {
    tunnel: [w103] -> w19
    tunnel: w4 -> [_]
    frame #0 {
      n18 = control-ref of="Tab Control"() -> (w103:refnum<vi>)
    }
  }
  n19 = property class="TabCtl (strict)"(reference=w19) -> ("Pages"=w9:refnum<vi>[])  [unwired: 1 in, 2 out]
  n20 = Index Array(array=w9, index #1=2 ("index"), index #2=0 ("index")) -> (element #1=w15:refnum<vi>, element #2=w16:refnum<vi>)
  n21 = property class="Page"(reference=w16) -> ("DecosOnPage"=w13:refnum<vi>[])  [unwired: 1 in, 2 out]
  n22 = property class="Page"(reference=w15) -> (error out=w10:errorcluster, "DecosOnPage"=w14:refnum<vi>[])  [unwired: 1 in, 1 out]
  n23 = Close Reference(reference=w9, error in (no error)=w10) -> ()  [unwired: 1 out]
  n24 = Index Array(array=w14) -> (element=w11:refnum<vi>)  [unwired: 1 in]
  n25 = Index Array(array=w13) -> (element=w12:refnum<vi>)  [unwired: 1 in]
  n26 = control-ref of="Tools"() -> (w74:refnum<vi>)
  n27 = control-ref of="Glyphs"() -> (w52:refnum<vi>)
  n28 = control-ref of="Templates"() -> (w53:refnum<vi>)
  n29 = control-ref of="Glyphs"() -> (w54:refnum<vi>)
  n30 = control-ref of="Font"() -> (w31:refnum<vi>)
  n31 = control-ref of="Line Color"() -> (w72:refnum<vi>)
  n32 = control-ref of="Fill Color"() -> (w73:refnum<vi>)
  n33 = control-ref of="refreshGlyphs"() -> (w20:refnum<vi>)
  n34 = control-ref of="refreshTemplates"() -> (w21:refnum<vi>)
  n35 = control-ref of="Move Up"() -> (w49:refnum<vi>)
  n36 = control-ref of="Move Down"() -> (w50:refnum<vi>)
  n37 = control-ref of="Add Layer"() -> (w37:refnum<vi>)
  n38 = control-ref of="Remove Layer"() -> (w38:refnum<vi>)
  n39 = control-ref of="Body Text Spec"() -> (w46:refnum<vi>)
  n40 = control-ref of="Icon Text"() -> (w56:refnum<vi>)
  n41 = control-ref of="Icon Template"() -> (w57:refnum<vi>)
  n42 = control-ref of="Color icon in"() -> (w34:refnum<vi>)
  n43 = control-ref of="Color icon in"() -> (w61:refnum<vi>)
  n44 = control-ref of="User Layers"() -> (w63:refnum<vi>)
  n45 = control-ref of="Body Text"() -> (w65:refnum<vi>)
  n46 = control-ref of="Framework Templates"() -> (w68:refnum<vi>)
  n47 = control-ref of="Clipboard"() -> (w59:refnum<vi>)
  n48 = control-ref of="Icon"() -> (w75:refnum<vi>)
  n49 = control-ref of="Preview"() -> (w76:refnum<vi>)
  n50 = control-ref of="Preview2"() -> (w45:refnum<vi>)
  n51 = control-ref of="Terminals"() -> (w64:refnum<vi>)
  n52 = control-ref of="IE VI Ref"() -> (w51:refnum<vi>)
  n53 = control-ref of="LayerName"() -> (w25:refnum<vi>)
  n54 = control-ref of="LayerName"() -> (w26:refnum<vi>)
  n55 = control-ref of="LayerName"() -> (w27:refnum<vi>)
  n56 = control-ref of="LayerName"() -> (w28:refnum<vi>)
  n57 = control-ref of="Line 3 text"() -> (w42:refnum<vi>)
  n58 = control-ref of="Line 4 text"() -> (w43:refnum<vi>)
  n59 = control-ref of="glyph path str"() -> (w47:refnum<vi>)
  n60 = control-ref of="templates path str"() -> (w48:refnum<vi>)
  n61 = control-ref of="Filter templates by keyword"() -> (w69:refnum<vi>)
  n62 = control-ref of="TextMarker"() -> (w70:refnum<vi>)
  n63 = control-ref of="Filter glyphs by keyword"() -> (w71:refnum<vi>)
  n64 = control-ref of="Line 1 text"() -> (w40:refnum<vi>)
  n65 = control-ref of="Line 2 text"() -> (w41:refnum<vi>)
  n66 = control-ref of="Glyphs []"() -> (w35:refnum<vi>)
  n67 = Current VI's Menubar() -> (w62:refnum<k9>)
  n68 = Build Array(w40, w41, w42, w43) -> (w39:refnum<vi>[])
  n69 = Build Array(w25, w26, w27, w28) -> (w23:refnum<vi>[])
  n70 = property on="OK" class="Bool"("KeyNav"=T24 {"Control"=FALSE, "Shift"=FALSE, "Key"="<Return>"} ("Key Navigation")) -> (error out=w32:errorcluster)  [unwired: 2 in, 1 out]
  n71 = Bundle(cluster=T23 {"Add Layer"=refnum, "Remove Layer"=refnum, "Line Text"=[], "Body Text Spec"=refnum, "DNL_Font"=refnum, "glyph path str"=refnum, "templates path str"=refnum, "Arrow Up"=refnum, "Arrow Down"=refnum, "IE VI Ref"=refnum, "Glyphs tree"=refnum, "Templates tree"=refnum, "Layer Icon Text"=refnum, "Layer Template"=refnum, "Clipboard"=refnum, "BW icon in"=refnum, "Color icon in"=refnum, "Layer Clust"=refnum, "Body Text"=refnum, "DNL_Framework Templates"=refnum, "Search Templates"=refnum, "TextMarker"=refnum, "Tab Control"=refnum, "Search Glyphs"=refnum, "Line Color"=refnum, "DNL_Glyphs []"=refnum, "Fill Color"=refnum, "Tools"=refnum, "Glyphs tree"=refnum, "Icon"=refnum, "Preview"=refnum, "Ants"=refnum, "Terminals"=refnum, "menu reference"=refnum, "LayerNames"=[], "GlyphLoadAnimation"=refnum, "TemplateLoadAnimation"=refnum, "refreshGlyphs"=refnum, "refreshTemplates"=refnum} ("references"), "Add Layer"=w37, "Remove Layer"=w38, "Line Text"=w39, "Body Text Spec"=w46, "DNL_Font"=w31, "glyph path str"=w47, "templates path str"=w48, "Arrow Up"=w49, "Arrow Down"=w50, "IE VI Ref"=w51, "Glyphs tree"=w52, "Templates tree"=w53, "Layer Icon Text"=w56, "Layer Template"=w57, "Clipboard"=w59, "BW icon in"=w34, "Color icon in"=w61, "Layer Clust"=w63, "Body Text"=w65, "DNL_Framework Templates"=w68, "Search Templates"=w69, "TextMarker"=w70, "Tab Control"=w19, "Search Glyphs"=w71, "Line Color"=w72, "DNL_Glyphs []"=w35, "Fill Color"=w73, "Tools"=w74, "Glyphs tree"=w54, "Icon"=w75, "Preview"=w76, "Ants"=w45, "Terminals"=w64, "menu reference"=w62, "LayerNames"=w23, "GlyphLoadAnimation"=w11, "TemplateLoadAnimation"=w12, "refreshGlyphs"=w20, "refreshTemplates"=w21) -> (w24:T23)
  n72 = call "NIIE_Initialization_UserEvents.vi"("Error"=w32, "Refs"=w24) -> ("Error Out"=w58:errorcluster, "Events Out"=w67:refnum<event-registration>, "User Events Out"=w1:T27)  [unwired: 7 out]
  n73 = Bundle("Events Out"=w67) -> (w66:cluster{"Events Out":refnum<event-registration>})  [unwired: 1 in]
  n74 = call "NIIE_Classes Initialization.vi"("LabVIEW Icon"="LabVIEW Icon in", "Error"=w58, "User Events"=w1, "Ref Cluster"=w24) -> ("Error Out"=w8:errorcluster, "Data Out"=w44:T28)  [unwired: 1 in, 5 out]
  n75 = flat-sequence {
    tunnel: w8 -> [w104]
    tunnel: w3 -> [_]
    frame #0 {
      n76 = invoke class="VI" method="FP.Open"(error in=w104, "Activate"=FALSE ("Activate?")) -> ()  [unwired: 3 in, 5 out]
    }
  }
  n77 = case shown="No Error" w8 {
    selector: w8 -> [w122 w823]
    tunnel: w66 -> [w139 _]
    tunnel: [w137 w824] -> w60
    tunnel: [w134 _] -> w55
    tunnel: w1 -> [w128 _]
    tunnel: w44 -> [w127 _]
    tunnel: w24 -> [w125 _]
    tunnel: [w124 _] -> w36
    tunnel: "LabVIEW Icon in" -> [w117 w822]
    tunnel: [w120 w822] -> w29
    tunnel: w1 -> [w113 _]
    tunnel: w3 -> [w112 _]
    tunnel: w2 -> [w108 _]
    frame No Error {
      # "Make sure the Keep IE in Memory VI runs and completes before the main Icon Editor panel is closed."
      # "Running ants"
      n78 = Unbundle By Name(w127) -> ("Class.Ants"=w126:refnum<class "Ants.lvclass">)
      n79 = Obtain Queue(max queue size (-1, unlimited)=100, element data type=T33 {"Left"=0, "Top"=0} ("Origin"), error in (no error)=w122) -> (queue out=w129:refnum<queue>, error out=w130:errorcluster)  [unwired: 1 in, 2 out]
      n80 = call "NIIE_Buffer for lossless tracking.vi"("Ref Cluster"=w125, "User Events"=w128, "Error"=w130, "Buffer"=w129) -> ()  [unwired: 8 out]
      n81 = while {
        shift-right: [w149] -> w119
        shift-left: w122 -> [w157]
        tunnel: [w153] -> w140
        tunnel: w139 -> [w152]
        tunnel: [w151] -> w136
        tunnel: w129 -> [w146]
        tunnel: w128 -> [w145]
        shift-right: [w142] -> w121
        shift-left: w127 -> [w144]
        border: T31 {"Horizontal"=-1, "Vertical"=-1} ("Corrected Out") -> [_]
        tunnel: w113 -> [w141]
        stop <- w154 stop-if-true
        n82 = event shown="[2] Menu Selection (User);  Menu Selection (App)" {
          selector: w152 -> [_ _ _ _ _ _ _ _ _ _ _ _ _ _ _ _ _ _ _ _ _ _ _ _ _ _ _ _ _ _ _ _ _ _ _ _ _ _ _ _ _ _ _ _ _ _ _ _ _ _ _]
          dyn-events: [_ _ _ _ _ _ _ _ _ _ _ _ _ _ _ _ _ _ _ _ _ _ _ _ _ _ _ _ _ _ _ _ _ _ _ _ _ _ _ _ _ _ _ _ _ _ _ _ _ _ _] -> w153
          timeout: _ -> [_ _ _ _ _ _ _ _ _ _ _ _ _ _ _ _ _ _ _ _ _ _ _ _ _ _ _ _ _ _ _ _ _ _ _ _ _ _ _ _ _ _ _ _ _ _ _ _ _ _ _]
          tunnel: [w163 errorcluster {"status"=TRUE, "code"=43, "source"=""} ("error out") w179 w202 w220 w224 w244 w266 w282 w298 w302 w316 w334 w341 w351 w359 w369 w379 w395 w403 w422 w436 w444 w462 w477 w492 w509 w524 w536 w543 w561 w571 w582 w585 w594 w608 w617 w629 w646 w656 w667 w670 w679 w692 errorcluster {"status"=TRUE, "code"=43, "source"=""} ("error out") w716 w746 w762 w767 w774 w781] -> w150
          tunnel: w157 -> [w165 _ w181 w204 w222 w229 w256 w260 w283 w299 w305 w317 w335 w340 w350 w361 w372 w387 w399 w412 w429 w437 w449 w467 w480 w498 w521 w531 w536 w542 w562 w574 w582 w586 w603 w611 w620 w631 w650 w657 w667 w671 w683 w695 _ w722 w750 w763 w768 w775 w782]
          tunnel: [TRUE w172 _ _ _ _ _ _ _ _ _ _ _ _ _ _ _ _ _ _ _ _ _ _ _ _ _ _ _ _ _ _ _ _ _ _ _ _ _ _ _ _ _ _ w710 _ _ _ _ _ _] -> w155
          tunnel: "Tools" -> [_ _ w175 _ _ _ _ _ _ w297 _ _ _ _ _ _ _ _ _ _ _ _ _ _ _ _ _ _ _ _ _ _ _ _ _ _ _ _ _ _ _ _ _ _ _ _ _ _ _ _ _]
          tunnel: [TRUE w172 TRUE TRUE _ TRUE TRUE TRUE TRUE TRUE TRUE TRUE TRUE TRUE _ TRUE _ _ TRUE _ _ TRUE TRUE TRUE _ TRUE _ _ _ _ _ TRUE _ _ TRUE _ _ TRUE TRUE _ _ _ _ TRUE w710 TRUE ("Yes") TRUE _ _ _ _] -> w147
          tunnel: w146 -> [_ _ _ _ _ _ _ _ w280 _ _ _ _ _ _ _ _ _ _ _ _ _ _ _ _ _ _ _ _ _ _ _ _ _ _ _ _ _ _ _ _ _ _ _ _ _ _ _ _ _ _]
          tunnel: w145 -> [_ _ w178 _ _ _ _ _ _ _ _ _ _ _ _ _ _ _ _ _ _ _ _ _ _ _ _ _ _ _ _ _ _ _ _ _ _ _ _ _ _ _ _ _ _ _ _ _ _ _ _]
          tunnel: w144 -> [w162 w171 w177 w200 w219 w228 w252 w262 w279 w295 w301 w312 w331 w339 w349 w354 w365 w377 w391 w408 w427 w434 w440 w458 w475 w490 w513 w529 w535 w540 w553 w569 w580 w583 w590 w607 w616 w627 w649 w654 w664 w673 w685 w702 w712 w721 w743 w765 w769 w772 w779]
          tunnel: [w158 w171 w176 w198 w218 w233 w245 w265 w278 w293 w300 w309 w330 w337 w347 w355 w364 w381 w390 w404 w421 w433 w438 w456 w474 w489 w507 w525 w535 w538 w551 w568 w580 w584 w595 w606 w615 w621 w644 w653 w666 w673 w677 w688 w712 w714 w740 w764 w769 w772 w779] -> w143
          tunnel: [_ _ _ _ _ _ _ _ _ _ _ w306 _ _ _ _ _ _ _ _ _ _ _ _ _ _ _ _ _ _ _ _ _ _ _ _ _ _ _ _ _ _ _ _ _ _ _ _ _ _ _] -> _
          tunnel: w141 -> [_ _ _ _ _ _ _ _ _ _ _ _ _ _ _ _ _ _ _ _ _ _ _ _ _ _ _ _ _ _ _ _ _ _ _ _ _ _ _ _ _ _ _ _ _ _ _ _ _ w773 w780]
          event "OK": Value Change {
            n83 = event-data() -> ()  [unwired: 2 out]
            n84 = call "NIIE_Finalize Text.vi"("Error"=w165, "Data"=w162) -> ("Error Out"=w166:errorcluster, "Data Out"=w161:T28)  [unwired: 8 out]
            n85 = call "NIIE_Finalize Movement.vi"("Error"=w166, "Data"=w161) -> ("Error Out"=w167:errorcluster, "Data Out"=w160:T28)  [unwired: 1 in, 7 out]
            n86 = call "NIIE_Layer_Deselect.vi"("Error"=w167, "Data"=w160) -> ("Error Out"=w164:errorcluster, "Data Out"=w159:T28)  [unwired: 8 out]
            n87 = call "NIIE_Reset layer template selection.vi"("Error"=w164, "Data"=w159) -> ("Error Out"=w163:errorcluster, "Data Out"=w158:T28)  [unwired: 1 in, 7 out]
          }
          event "Cancel": Value Change {
            w172 = FALSE ("Yes")
            n88 = event-data() -> ()  [unwired: 2 out]
          }
          event Menu Selection (User); Menu Selection (App) {
            n89 = event-data() -> ("Type"=w182:T35, "ItemTag"=w183:string)  [unwired: 1 out]
            n90 = case shown="\"Text\"" w175 {
              tunnel: w181 -> [w184 w189]
              tunnel: w177 -> [w185 w188]
              tunnel: [w184 w187] -> w173
              tunnel: [w185 w186] -> w174
              frame Default {
              }
              frame "Text" {
                n91 = call "NIIE_Finalize Text.vi"("Error"=w189, "Data"=w188) -> ("Error Out"=w187:errorcluster, "Data Out"=w186:T28)  [unwired: 8 out]
              }
            }
            n92 = case shown="\"Menu Selection (User)\"" w182 {
              tunnel: w183 -> [_ w197]
              tunnel: [w191 w196] -> w179
              tunnel: w173 -> [w191 w195]
              tunnel: w178 -> [_ w194]
              tunnel: w174 -> [w190 w193]
              tunnel: [w190 w192] -> w176
              frame Default {
              }
              frame "Menu Selection (User)" {
                n93 = call "NIIE_MenuSelection(User).vi"("User Events"=w194, "Error"=w195, "ItemTag"=w197, "Data"=w193) -> ("Error Out"=w196:errorcluster, "Data Out"=w192:T28)  [unwired: 1 in, 5 out]
              }
            }
          }
          event Mouse Down {
            n94 = event-data() -> ("CtlRef"=w203:refnum<vi>, "Button"=w199:u16)  [unwired: 1 out]
            n95 = case shown="1, 2" w199 {
              tunnel: w204 -> [w206 w213]
              tunnel: w203 -> [_ w217]
              tunnel: [w206 w211] -> w202
              tunnel: w200 -> [w205 w208]
              tunnel: [w205 w207] -> w198
              frame 0, Default {
              }
              frame 1, 2 {
                n96 = control-ref of="This VI"() -> (w216:refnum<vi>)
                n97 = call "NIIE_Defer_FP_Updates.vi"("Defer Panel Updates"=TRUE, "error in (no error)"=w213, "lv_icon.vi in"=w216) -> ("error out"=w214:errorcluster, "lv icon.vi out"=w209:refnum<vi>)  [unwired: 7 out]
                n98 = call "NIIE_Template_MouseDown.vi"("Add To Undo?"=TRUE ("Add to Undo?"), "Error"=w214, "CtlRef"=w217, "Data"=w208) -> ("Error Out"=w212:errorcluster, "Data Out"=w207:T28)  [unwired: 1 in, 5 out]
                n99 = call "NIIE_Defer_FP_Updates.vi"("error in (no error)"=w212, "lv_icon.vi in"=w209) -> ("error out"=w211:errorcluster)  [unwired: 1 in, 8 out]
              }
            }
          }
          event Value Change {
            n100 = event-data() -> ("NewVal"=w221:T21)  [unwired: 1 out]
            n101 = call "NIIE_Value Change_Tools.vi"("Error"=w222, "NewVal"=w221, "Data"=w219) -> ("Error Out"=w220:errorcluster, "Data Out"=w218:T28)  [unwired: 7 out]
          }
          event Mouse Down {
            n102 = event-data() -> ("Mods.Double Click"=w223:bool)  [unwired: 1 out]
            n103 = call "NIIE_Finalize Text.vi"("Error"=w229, "Data"=w228) -> ("Error Out"=w231:errorcluster, "Data Out"=w230:T28)  [unwired: 8 out]
            n104 = call "NIIE_Finalize Movement.vi"("Error"=w231, "Data"=w230) -> ("Error Out"=w227:errorcluster, "Data Out"=w226:T28)  [unwired: 1 in, 7 out]
            n105 = call "NIIE_Mouse Down.vi"("Error"=w227, "Double Click"=w223, "Data"=w226) -> ("Error Out"=w224:errorcluster, "Data Out"=w225:T28)  [unwired: 7 out]
            n106 = Bundle By Name(cluster=w225, "Support.Tool (old value)"=u32 111) -> (w233:T28)
          }
          event Value Change {
            # "Body Text Value Change event is fired programmatically during initialization so first call of this event is guaranteed to be a case we do not want to update the undo/redo information."
            n107 = event-data() -> ("OldVal"=w243:T8, "NewVal"=w242:T8, "OldVal.Body Text Spec.Alignment"=w247:T10)  [unwired: 1 out]
            n108 = local read "Tab Control"() -> (w238:T5)
            n109 = Unbundle By Name(w243) -> ("Body Text Spec.Font"=w241:T9)
            n110 = First Call?() -> (First Call?: T/F=w255:bool)
            n111 = Equal?(x=w238, y=T5."Icon Text") -> (x = y?=w236:bool)
            n112 = Not(x=w255) -> (.not. x?=w254:bool)
            n113 = Unbundle By Name(w242) -> ("Body Text Spec.Font"=w240:T9)
            n114 = Unbundle By Name(w242) -> ("Body Text Spec.Alignment"=w248:T10)
            n115 = Not Equal?(x=w241, y=w240) -> (x != y?=w239:bool)
            n116 = And(x=w236, y=w239) -> (x .and. y?=w235:bool)
            n117 = call "NIIE_Value Change_Body Text.vi"("Layer Icon"="Icon Text", "Add To Undo?"=w254, "Error"=w256, "NewVal"=w242, "Data"=w252) -> ("Error Out"=w250:errorcluster, "Data Out"=w249:T28)  [unwired: 5 out]
            n118 = case shown="True" w235 {
              frame False {
              }
              frame True {
                n119 = property on="Line 1 text" class="Str"("Key Focus"=TRUE) -> ()  [unwired: 2 in, 2 out]
              }
            }
            n120 = Not Equal?(x=w248, y=w247) -> (x != y?=w246:bool)
            n121 = call "NIIE_Alignment Value Change.vi"("Set Focus?"=w246, "Error"=w250, "NewVal"=w248, "Data"=w249) -> ("Error Out"=w244:errorcluster, "Data Out"=w245:T28)  [unwired: 6 out]
          }
          event Value Change {
            n122 = event-data() -> ()  [unwired: 2 out]
            n123 = call "NIIE_Finalize Text.vi"("Error"=w260, "Data"=w262) -> ("Error Out"=w264:errorcluster, "Data Out"=w263:T28)  [unwired: 8 out]
            n124 = local read "Line Color"() -> (w259:T20)
            n125 = local read "Fill Color"() -> (w269:T20)
            n126 = call "NIIE_Finalize Movement.vi"("Error"=w264, "Data"=w263) -> ("Error Out"=w258:errorcluster, "Data Out"=w261:T28)  [unwired: 1 in, 7 out]
            n127 = stacked-sequence {
              tunnel: w269 -> [w273]
              tunnel: [w272] -> w267
              tunnel: w259 -> [w271]
              tunnel: w258 -> [w270]
              frame #0 {
                n128 = local write "Fill Color"(w271) -> ()
                n129 = property on="Line Color" class="ColBox (strict)"(error in=w270, "Val(Sgnl)"=w273) -> (error out=w272:errorcluster)  [unwired: 1 in, 1 out]
              }
            }
            n130 = call "NIIE_Escape.vi"("Error"=w267, "Data"=w261) -> ("Error Out"=w266:errorcluster, "Data Out"=w265:T28)  [unwired: 1 in, 7 out]
          }
          event "Preview", "Terminals", "Preview2": Mouse Move {
            n131 = event-data() -> ("Coords"=w277:T31)  [unwired: 1 out]
            n132 = call "NIIE_CoordinatesCorrection.vi"("Coordinates In"=w277) -> ("Corrected Out"=w274:T31)  [unwired: 10 out]
            n133 = feedback-in #1(w274) -> ()
            n134 = feedback #1() -> (w276:T31)
            n135 = Not Equal?(x=w274, y=w276) -> (x != y?=w275:bool)
            n136 = case shown="True" w275 {
              tunnel: w283 -> [w285 w291]
              tunnel: [w285 w290] -> w282
              tunnel: w280 -> [_ w289]
              tunnel: w279 -> [w284 w288]
              tunnel: [w284 w287] -> w278
              tunnel: w274 -> [_ w286]
              frame False {
              }
              frame True {
                n137 = call "NIIE_MouseMove.vi"("Buffer"=w289, "Error"=w291, "Coords"=w286, "Data"=w288) -> ("Error Out"=w290:errorcluster, "Data Out"=w287:T28)  [unwired: 6 out]
              }
            }
          }
          event "Preview", "Terminals", "Preview2": Mouse Enter {
            n138 = event-data() -> ()  [unwired: 2 out]
            n139 = call "NIIE_SetCursor.vi"("Error"=w299, "Radio Buttons"=w297, "Data"=w295) -> ("Error Out"=w298:errorcluster, "Data Out"=w294:T28)  [unwired: 7 out]
            n140 = Bundle By Name(cluster=w294, "Support.Mouse inside icon?"=TRUE) -> (w293:T28)
          }
          event "Preview", "Terminals", "Preview2": Mouse Up {
            n141 = event-data() -> ("Coords"=w304:T31)  [unwired: 1 out]
            n142 = call "NIIE_PictureControl_MouseUp.vi"("Error"=w305, "Coords"=w304, "Data"=w301) -> ("Error Out"=w302:errorcluster, "Data Out"=w300:T28)  [unwired: 4 in, 3 out]
          }
          event Key Down?; event type 5.0.x8000000b {
            n143 = event-data() -> ("Type"=w311:T35, "Char"=w308:i16, "VKey"=w315:T36, "PlatMods"=w310:T37)  [unwired: 1 out]
            n144 = Equal?(x=i16 99, y=w308) -> (x = y?=w306:bool)
            n145 = call "NIIE_KeyDown.vi"("PlatMods"=w310, "Type"=w311, "Error"=w317, "VKey"=w315, "Char"=w308, "Data"=w312) -> ("Error Out"=w316:errorcluster, "Discard? Out"=w314:bool, "Data Out"=w309:T28)  [unwired: 3 out]
            n146 = event-data("Discard?"=w314) -> ()  [unwired: 1 in, 1 out]
          }
          event "Preview", "Terminals", "Preview2": Mouse Down {
            # "Left click"
            n147 = event-data() -> ("Button"=w320:u16, "Coords"=w333:T31)  [unwired: 1 out]
            n148 = Not Equal?(x=u16 1, y=w320) -> (x != y?=w318:bool)
            n149 = control-ref of="This VI"() -> (w329:refnum<vi>)
            n150 = call "NIIE_Defer_FP_Updates.vi"("Defer Panel Updates"=TRUE, "error in (no error)"=w335, "lv_icon.vi in"=w329) -> ("error out"=w325:errorcluster, "lv icon.vi out"=w327:refnum<vi>)  [unwired: 7 out]
            n151 = call "NIIE_Reset layer template selection.vi"("Force Reset? (T)"=FALSE ("Force reset? (T)"), "Error"=w325, "Data"=w331) -> ("Error Out"=w324:errorcluster, "Data Out"=w321:T28)  [unwired: 1 in, 6 out]
            n152 = call "NIIE_MouseDown.vi"("Flip Colors?"=w318, "Error"=w324, "Coords"=w333, "Data"=w321) -> ("Error Out"=w323:errorcluster, "Data Out"=w330:T28)  [unwired: 1 in, 5 out]
            n153 = call "NIIE_Defer_FP_Updates.vi"("Defer Panel Updates"=FALSE, "error in (no error)"=w323, "lv_icon.vi in"=w327) -> ("error out"=w334:errorcluster)  [unwired: 8 out]
          }
          event Value Change {
            n154 = event-data() -> ()  [unwired: 2 out]
            n155 = call "Check Color.vi"("Color in"="Fill Color") -> ("Color out"=w342:T20)  [unwired: 10 in]
            n156 = call "Check Color.vi"("Color in"="Line Color") -> ("Color out"=w343:T20)  [unwired: 10 in]
            n157 = Bundle By Name(cluster=w339, "Support.Fill Color"=w342, "Support.Edge Color"=w343) -> (w338:T28)
            n158 = call "NIIE_Escape.vi"("Reset Cursor (T)"=FALSE ("Reset cursor? (T)"), "Error"=w340, "Data"=w338) -> ("Error Out"=w341:errorcluster, "Data Out"=w337:T28)  [unwired: 1 in, 6 out]
          }
          event Key Up {
            n159 = event-data() -> ("PlatMods"=w348:T37)  [unwired: 1 out]
            n160 = call "NIIE_KeyUp.vi"("Error"=w350, "PlatMods"=w348, "Data"=w349) -> ("Error Out"=w351:errorcluster, "Data Out"=w347:T28)  [unwired: 7 out]
          }
          event Value Change {
            n161 = event-data() -> ()  [unwired: 2 out]
            n162 = call "NIIE_Finalize Text.vi"("Error"=w361, "Data"=w354) -> ("Error Out"=w360:errorcluster, "Data Out"=w356:T28)  [unwired: 8 out]
            n163 = call "NIIE_Finalize Movement.vi"("Error"=w360, "Data"=w356) -> ("Error Out"=w357:errorcluster, "Data Out"=w353:T28)  [unwired: 1 in, 7 out]
            n164 = call "NIIE_RotateFlip.vi"("Error"=w357, "Rotate"="Clockwise Rotate", "Data"=w353) -> ("Error Out"=w358:errorcluster, "Data Out"=w352:T28)  [unwired: 2 in, 5 out]
            n165 = call "NIIE_Escape.vi"("Error"=w358, "Data"=w352) -> ("Error Out"=w359:errorcluster, "Data Out"=w355:T28)  [unwired: 1 in, 7 out]
          }
          event Value Change {
            n166 = event-data() -> ("NewVal"=w374:variant)  [unwired: 1 out]
            n167 = control-ref of="This VI"() -> (w371:refnum<vi>)
            n168 = call "NIIE_Defer_FP_Updates.vi"("Defer Panel Updates"=TRUE, "error in (no error)"=w372, "lv_icon.vi in"=w371) -> ("error out"=w373:errorcluster, "lv icon.vi out"=w366:refnum<vi>)  [unwired: 7 out]
            n169 = call "NIIE_Mouse Down_Templates.vi"("Tag"="Templates", "Error"=w373, "NewVal"=w374, "Data"=w365) -> ("Error Out"=w368:errorcluster, "Data Out"=w364:T28)  [unwired: 1 in, 5 out]
            n170 = call "NIIE_Defer_FP_Updates.vi"("error in (no error)"=w368, "lv_icon.vi in"=w366) -> ("error out"=w369:errorcluster)  [unwired: 1 in, 8 out]
          }
          event User Event {
            # "This is an initialization event for the glyphs."
            n171 = event-data() -> ("Glyphs"=w389:string)  [unwired: 1 out]
            n172 = Unbundle By Name(w377) -> ("Ref.GlyphLoadAnimation"=w376:refnum<vi>, "Ref.refreshGlyphs"=w375:refnum<vi>)
            n173 = Unflatten From String(type="?", binary string=w389, error in (no error)=w387) -> (value=w384:T3[], error out=w386:errorcluster)  [unwired: 3 out]
            n174 = call "NIIE_Populate Graphics.vi"("Error"=w386, "Glyphs []"=w384, "Data"=w377) -> ("Error Out"=w385:errorcluster, "Data Out"=w381:T28)  [unwired: 7 out]
            n175 = call "File_Write Glyphs to Binary File.vi"("File Name"="Glyphs.bin", "Path"=Pathes."Glyphs", "Error"=w385, "Graphics []"=w384) -> ("Error Out"=w380:errorcluster)  [unwired: 7 out]
            n176 = call "NIIE_ChangeRefreshGraphicsState.vi"("error in (no error)"=w380, "refreshing?"=FALSE, "button ref"=w375, "animatedDecoration ref"=w376) -> ("error out"=w379:errorcluster)  [unwired: 7 in]
          }
          event Mouse Down {
            n177 = event-data() -> ("PlatMods.Shift"=w392:bool, "CtlRef"=w402:refnum<vi>, "PlatMods.Ctrl"=w401:bool)  [unwired: 1 out]
            n178 = control-ref of="This VI"() -> (w398:refnum<vi>)
            n179 = call "NIIE_Defer_FP_Updates.vi"("Defer Panel Updates"=TRUE, "error in (no error)"=w399, "lv_icon.vi in"=w398) -> ("error out"=w397:errorcluster, "lv icon.vi out"=w394:refnum<vi>)  [unwired: 7 out]
            n180 = call "NIIE_Mouse Down_User Layers.vi"("Shift"=w392, "Error"=w397, "Ctrl"=w401, "CtlRef"=w402, "Data"=w391) -> ("Error Out"=w396:errorcluster, "Data Out"=w390:T28)  [unwired: 5 out]
            n181 = call "NIIE_Defer_FP_Updates.vi"("error in (no error)"=w396, "lv_icon.vi in"=w394) -> ("error out"=w395:errorcluster)  [unwired: 1 in, 8 out]
          }
          event "Filter glyphs by keyword": Mouse Down {
            # "If a mouse down event should\nselect the entered text, enable this case"
            n182 = event-data() -> ("CtlRef"=w411:refnum<vi>)  [unwired: 1 out]
            n183 = disable-structure shown="Enabled" {
              disable-tunnel: w412 -> [w415 w418]
              disable-tunnel: w411 -> [w414 _]
              disable-tunnel: [w413 w418] -> w410
              frame Disabled {
                n184 = property class="Str"(reference=w414, error in=w415, "Text.Selection Start"=u32 0 ("Text.Selection:Start"), "Text.Selection End"=-1 ("Text.Selection:End")) -> (error out=w413:errorcluster)  [unwired: 1 out]
              }
              frame Enabled {
              }
            }
            n185 = call "NIIE_Finalize Text.vi"("Error"=w410, "Data"=w408) -> ("Error Out"=w409:errorcluster, "Data Out"=w407:T28)  [unwired: 8 out]
            n186 = call "NIIE_Layer_Deselect.vi"("Error"=w409, "Data"=w407) -> ("Error Out"=w406:errorcluster, "Data Out"=w405:T28)  [unwired: 8 out]
            n187 = call "NIIE_Escape.vi"("Error"=w406, "Data"=w405) -> ("Error Out"=w403:errorcluster, "Data Out"=w404:T28)  [unwired: 1 in, 7 out]
          }
          event "Filter glyphs by keyword": Value Change {
            n188 = event-data() -> ("NewVal"=w432:string)  [unwired: 1 out]
            n189 = Unbundle By Name(w427) -> ("Class.Glyph"=w428:refnum<class "Glyph.lvclass">, "Ref.DNL_Glyphs []"=w425:refnum<vi>, "Ref.Glyphs tree"=w424:refnum<vi>)
            n190 = First Call?() -> (First Call?: T/F=w430:bool)
            n191 = Not(x=w430) -> (.not. x?=w431:bool)
            n192 = call "SearchGlyphs.vi"("Glyphs Tree"=w424, "DNL_Glyphs []"=w425, "Reset Position? (F)"=w431, "Error"=w429, "Keyword"=w432, "Glyph"=w428) -> ("Error Out"=w423:errorcluster, "Glyph Out"=w426:refnum<class "Glyph.lvclass">)  [unwired: 4 out]
            n193 = Bundle By Name(cluster=w427, "Class.Glyph"=w426) -> (w420:T28)
            n194 = call "NIIE_Undo_Add Data to History.vi"("Add To Undo?"=TRUE ("Add to Undo?"), "Error"=w423, "Data"=w420) -> ("Error Out"=w422:errorcluster, "Data Out"=w421:T28)  [unwired: 7 out]
          }
          event Mouse Down {
            n195 = event-data() -> ()  [unwired: 2 out]
            n196 = call "NIIE_MouseDown_Body Text.vi"("Error"=w437, "Data"=w434) -> ("Error Out"=w436:errorcluster, "Data Out"=w433:T28)  [unwired: 8 out]
          }
          event Value Change {
            n197 = event-data() -> ("OldVal.Opacity"=w443:u8, "NewVal.Opacity"=w442:u8, "NewVal"=w448:T15)  [unwired: 1 out]
            n198 = Not Equal?(x=w443, y=w442) -> (x != y?=w441:bool)
            n199 = call "NIIE_Value Change_Top or Bottom Layer.vi"("Type"=enum16{"Template Layer", "Text Layer"}."Text Layer", "Error"=w449, 10:"Data"=w448, 11:"Data"=w440) -> ("Error Out"=w445:errorcluster, "Data Out"=w439:T28)  [unwired: 6 out]
            n200 = case shown="True" w441 {
              tunnel: w445 -> [w451 w455]
              tunnel: [w451 w454] -> w444
              tunnel: w439 -> [w450 w453]
              tunnel: [w450 w452] -> w438
              frame False {
              }
              frame True {
                n201 = call "NIIE_Reset layer template selection.vi"("Error"=w455, "Data"=w453) -> ("Error Out"=w454:errorcluster, "Data Out"=w452:T28)  [unwired: 1 in, 7 out]
              }
            }
          }
          event Value Change {
            n202 = event-data() -> ("OldVal.Opacity"=w460:u8, "NewVal.Opacity"=w461:u8, "NewVal"=w465:T15)  [unwired: 1 out]
            n203 = Not Equal?(x=w460, y=w461) -> (x != y?=w459:bool)
            n204 = call "NIIE_Value Change_Top or Bottom Layer.vi"("Type"=enum16{"Template Layer", "Text Layer"}."Template Layer", "Error"=w467, 10:"Data"=w465, 11:"Data"=w458) -> ("Error Out"=w463:errorcluster, "Data Out"=w457:T28)  [unwired: 6 out]
            n205 = case shown="True" w459 {
              tunnel: w463 -> [w469 w473]
              tunnel: [w469 w472] -> w462
              tunnel: w457 -> [w468 w471]
              tunnel: [w468 w470] -> w456
              frame False {
              }
              frame True {
                n206 = call "NIIE_Reset layer template selection.vi"("Error"=w473, "Data"=w471) -> ("Error Out"=w472:errorcluster, "Data Out"=w470:T28)  [unwired: 1 in, 7 out]
              }
            }
          }
          event Value Change {
            n207 = event-data() -> ("NewVal"=w484:variant)  [unwired: 1 out]
            n208 = control-ref of="This VI"() -> (w481:refnum<vi>)
            n209 = call "NIIE_Defer_FP_Updates.vi"("Defer Panel Updates"=TRUE, "error in (no error)"=w480, "lv_icon.vi in"=w481) -> ("error out"=w479:errorcluster, "lv icon.vi out"=w476:refnum<vi>)  [unwired: 7 out]
            n210 = Variant To Data(error in=w479, type=0, Variant=w484) -> (data=w483:i32, error out=w485:errorcluster)
            n211 = call "NIIE_UpdateLayerView_ScrollbarChanged.vi"("Error"=w485, "Scrollbar Position"=w483, "Data"=w475) -> ("Error Out"=w478:errorcluster, "Data Out"=w474:T28)  [unwired: 7 out]
            n212 = call "NIIE_Defer_FP_Updates.vi"("error in (no error)"=w478, "lv_icon.vi in"=w476) -> ("error out"=w477:errorcluster)  [unwired: 1 in, 8 out]
          }
          event Value Change {
            # "We do not use the dynamic registerd event for Layer Clust.Value Change\nbecause it would be a huge effort to lock the front panel until this\nevent case has been completed."
            n213 = event-data() -> ("OldVal.Visibility?"=w488:bool, "CtlRef"=w502:refnum<vi>, "OldVal.LayerName"=w487:string)  [unwired: 1 out]
            n214 = control-ref of="This VI"() -> (w499:refnum<vi>)
            n215 = call "NIIE_Defer_FP_Updates.vi"("Defer Panel Updates"=TRUE, "error in (no error)"=w498, "lv_icon.vi in"=w499) -> ("error out"=w497:errorcluster, "lv icon.vi out"=w494:refnum<vi>)  [unwired: 7 out]
            n216 = call "NIIE_LayerCluster_ValueChange.vi"("Old Visibility?"=w488, "Error"=w497, "Old Name"=w487, "CtlRef"=w502, "Data"=w490) -> ("Error Out"=w496:errorcluster, "Data Out"=w491:T28)  [unwired: 1 in, 4 out]
            n217 = call "NIIE_Defer_FP_Updates.vi"("Defer Panel Updates"=FALSE, "error in (no error)"=w496, "lv_icon.vi in"=w494) -> ("error out"=w493:errorcluster)  [unwired: 8 out]
            n218 = call "NIIE_Reset layer template selection.vi"("Error"=w493, "Data"=w491) -> ("Error Out"=w492:errorcluster, "Data Out"=w489:T28)  [unwired: 1 in, 7 out]
          }
          event "Filter templates by keyword": Value Change {
            n219 = event-data() -> ("NewVal"=w505:string)  [unwired: 1 out]
            n220 = Unbundle By Name(w513) -> ("Ref.Templates tree"=w506:refnum<vi>, "Class.Templates"=w514:refnum<class "FakedArray.lvclass">)
            n221 = control-ref of="This VI"() -> (w523:refnum<vi>)
            n222 = call "NIIE_Defer_FP_Updates.vi"("Defer Panel Updates"=TRUE, "error in (no error)"=w521, "lv_icon.vi in"=w523) -> ("error out"=w516:errorcluster, "lv icon.vi out"=w520:refnum<vi>)  [unwired: 7 out]
            n223 = call-dynamic "SET_ScrollbarPosition.vi"("error in (no error)"=w516, "FakedArray.lvclass in"=w514) -> ("error out"=w517:errorcluster, "FakedArray.lvclass out"=w518:refnum<class "FakedArray.lvclass">)  [unwired: 1 in, 7 out]
            n224 = call "ResetColor.vi"("error in (no error)"=w517, "FakedArray in"=w518) -> ("error out"=w504:errorcluster, "FakedArray out"=w519:refnum<class "FakedArray.lvclass">)  [unwired: 8 out]
            n225 = call "NIIE_Tree Set All.vi"("Error"=w504, "Value"=w505, "TreeControl"=w506) -> ("Error Out"=w503:errorcluster)  [unwired: 7 in, 1 out]
            n226 = call-dynamic "UpdateVisibleData.vi"("Error"=w503, "Keyword"=w505, "FakedArray"=w519) -> ("Error Out"=w515:errorcluster, "FakedArray Out"=w512:refnum<class "FakedArray.lvclass">)  [unwired: 2 in, 5 out]
            n227 = Bundle By Name(cluster=w513, "Class.Templates"=w512) -> (w508:T28)
            n228 = call "NIIE_Defer_FP_Updates.vi"("error in (no error)"=w515, "lv_icon.vi in"=w520) -> ("error out"=w510:errorcluster)  [unwired: 1 in, 8 out]
            n229 = call "NIIE_Undo_Add Data to History.vi"("Add To Undo?"=TRUE ("Add to Undo?"), "Error"=w510, "Data"=w508) -> ("Error Out"=w509:errorcluster, "Data Out"=w507:T28)  [unwired: 7 out]
          }
          event "Filter templates by keyword": Mouse Down {
            # "If a mouse down event should\nselect the entered text, enable this case"
            n230 = event-data() -> ()  [unwired: 2 out]
            n231 = call "NIIE_Finalize Text.vi"("Error"=w531, "Data"=w529) -> ("Error Out"=w530:errorcluster, "Data Out"=w528:T28)  [unwired: 8 out]
            n232 = call "NIIE_Layer_Deselect.vi"("Error"=w530, "Data"=w528) -> ("Error Out"=w527:errorcluster, "Data Out"=w526:T28)  [unwired: 8 out]
            n233 = call "NIIE_Escape.vi"("Error"=w527, "Data"=w526) -> ("Error Out"=w524:errorcluster, "Data Out"=w525:T28)  [unwired: 1 in, 7 out]
          }
          event "Help": Value Change {
            n234 = event-data() -> ()  [unwired: 2 out]
            n235 = control-ref of="This VI"() -> (w534:refnum<vi>)
            n236 = property class="VI"(reference=w534) -> (error out=w532:errorcluster, "Help.URL"=w533:string)  [unwired: 1 in, 1 out]
            n237 = call "NIIE_Open Help Link.vi"("error in (no error)"=w532, "Help.URL"=w533) -> ()  [unwired: 9 in, 1 out]
          }
          event "Glyphs": Value Change {
            n238 = event-data() -> ("NewVal"=w544:string)  [unwired: 1 out]
            n239 = Unbundle By Name(w540) -> ("Class.Glyph"=w541:refnum<class "Glyph.lvclass">, "Ref.DNL_Glyphs []"=w537:refnum<vi>)
            n240 = call "FilterGlyphs.vi"("error in (no error)"=w542, "DNL_Glyphs []"=w537, "Tag"=w544, "Glyph in"=w541) -> ("error out"=w543:errorcluster, "Glyph out"=w539:refnum<class "Glyph.lvclass">)  [unwired: 6 out]
            n241 = Bundle By Name(cluster=w540, "Class.Glyph"=w539) -> (w538:T28)
          }
          event "Templates": Value Change {
            w545 = "" ("Value")
            n242 = event-data() -> ("CtlRef"=w549:refnum<vi>, "NewVal"=w546:string)  [unwired: 1 out]
            n243 = control-ref of="This VI"() -> (w564:refnum<vi>)
            n244 = Unbundle By Name(w553) -> ("Class.Templates"=w554:refnum<class "FakedArray.lvclass">)
            n245 = local write "Filter templates by keyword"("") -> ()
            n246 = call "NIIE_Defer_FP_Updates.vi"("Defer Panel Updates"=TRUE, "error in (no error)"=w562, "lv_icon.vi in"=w564) -> ("error out"=w556:errorcluster, "lv icon.vi out"=w560:refnum<vi>)  [unwired: 7 out]
            n247 = call-dynamic "SET_ScrollbarPosition.vi"("error in (no error)"=w556, "FakedArray.lvclass in"=w554) -> ("error out"=w558:errorcluster, "FakedArray.lvclass out"=w557:refnum<class "FakedArray.lvclass">)  [unwired: 1 in, 7 out]
            n248 = call "ResetColor.vi"("error in (no error)"=w558, "FakedArray in"=w557) -> ("error out"=w548:errorcluster, "FakedArray out"=w559:refnum<class "FakedArray.lvclass">)  [unwired: 8 out]
            n249 = call "NIIE_Tree Set All.vi"("Error"=w548, "Value"=w545, "TreeControl"=w549) -> ("Error Out"=w547:errorcluster)  [unwired: 7 in, 1 out]
            n250 = call-dynamic "UpdateVisibleData.vi"("Error"=w547, "Tag"=w546, "Keyword"=w545, "FakedArray"=w559) -> ("Error Out"=w555:errorcluster, "FakedArray Out"=w552:refnum<class "FakedArray.lvclass">)  [unwired: 1 in, 5 out]
            n251 = Bundle By Name(cluster=w553, "Class.Templates"=w552) -> (w551:T28)
            n252 = call "NIIE_Defer_FP_Updates.vi"("error in (no error)"=w555, "lv_icon.vi in"=w560) -> ("error out"=w561:errorcluster)  [unwired: 1 in, 8 out]
          }
          event Value Change {
            n253 = event-data() -> ()  [unwired: 2 out]
            n254 = control-ref of="This VI"() -> (w575:refnum<vi>)
            n255 = call "NIIE_Defer_FP_Updates.vi"("Defer Panel Updates"=TRUE, "error in (no error)"=w574, "lv_icon.vi in"=w575) -> ("error out"=w573:errorcluster, "lv icon.vi out"=w572:refnum<vi>)  [unwired: 7 out]
            n256 = call "NIIE_MoveLayers.vi"("Error"=w573, "Arrow Up"="Move Up", "Data"=w569) -> ("Error Out"=w565:errorcluster, "Data Out"=w568:T28)  [unwired: 7 out]
            n257 = stacked-sequence {
              tunnel: [w578] -> w566
              tunnel: w565 -> [w578]
              frame #0 {
                w579 = FALSE ("Arrow Down")
                n258 = local write "Move Down"(w579) -> ()
                n259 = local write "Move Up"(w579) -> ()
              }
            }
            n260 = call "NIIE_Defer_FP_Updates.vi"("Defer Panel Updates"=FALSE, "error in (no error)"=w566, "lv_icon.vi in"=w572) -> ("error out"=w571:errorcluster)  [unwired: 8 out]
          }
          event Shortcut Menu Activation? {
            n261 = event-data() -> ()  [unwired: 2 out]
            n262 = event-data("Discard?"=TRUE) -> ()  [unwired: 1 in, 1 out]
          }
          event Mouse Leave; Mouse Up {
            n263 = event-data() -> ()  [unwired: 2 out]
            n264 = call "NIIE_Undo_Add Data to History.vi"("Add To Undo?"=TRUE ("Add to Undo?"), "Error"=w586, "Data"=w583) -> ("Error Out"=w585:errorcluster, "Data Out"=w584:T28)  [unwired: 7 out]
          }
          event User Event {
            # "This is an initialization event for the templates"
            n265 = event-data() -> ("Templates"=w605:string)  [unwired: 1 out]
            n266 = Unbundle By Name(w590) -> ("Ref.TemplateLoadAnimation"=w589:refnum<vi>, "Ref.refreshTemplates"=w588:refnum<vi>)
            n267 = control-ref of="This VI"() -> (w600:refnum<vi>)
            n268 = call "NIIE_Defer_FP_Updates.vi"("Defer Panel Updates"=TRUE, "error in (no error)"=w603, "lv_icon.vi in"=w600) -> ("error out"=w598:errorcluster, "lv icon.vi out"=w597:refnum<vi>)  [unwired: 7 out]
            n269 = Unflatten From String(type="?", binary string=w605, error in (no error)=w598) -> (value=w596:cluster{T1[], i32, bool}, error out=w601:errorcluster)  [unwired: 3 out]
            n270 = call "NIIE_Process Template Graphics.vi"("Error"=w601, "Match Data"=w596, "Data"=w590) -> ("Error Out"=w593:errorcluster, "Data Out"=w595:T28)  [unwired: 7 out]
            n271 = call "NIIE_ChangeRefreshGraphicsState.vi"("error in (no error)"=w593, "refreshing?"=FALSE, "button ref"=w588, "animatedDecoration ref"=w589) -> ("error out"=w592:errorcluster)  [unwired: 7 in]
            n272 = call "NIIE_Defer_FP_Updates.vi"("error in (no error)"=w592, "lv_icon.vi in"=w597) -> ("error out"=w594:errorcluster)  [unwired: 1 in, 8 out]
          }
          event "Templates": Mouse Down {
            n273 = event-data() -> ("CtlRef"=w610:refnum<vi>, "Coords"=w612:T31)  [unwired: 1 out]
            n274 = call "NIIE_Mouse Down_Tree.vi"("Tree"=w610, "Error"=w611, "Coords"=w612) -> ("Error Out"=w609:errorcluster)  [unwired: 8 out]
            n275 = call "NIIE_Escape.vi"("Error"=w609, "Data"=w607) -> ("Error Out"=w608:errorcluster, "Data Out"=w606:T28)  [unwired: 1 in, 7 out]
          }
          event "Glyphs": Mouse Down {
            n276 = event-data() -> ("CtlRef"=w614:refnum<vi>, "Coords"=w619:T31)  [unwired: 1 out]
            n277 = local write "Filter glyphs by keyword"("") -> ()
            n278 = call "NIIE_Mouse Down_Tree.vi"("Tree"=w614, "Error"=w620, "Coords"=w619) -> ("Error Out"=w618:errorcluster)  [unwired: 8 out]
            n279 = call "NIIE_Escape.vi"("Error"=w618, "Data"=w616) -> ("Error Out"=w617:errorcluster, "Data Out"=w615:T28)  [unwired: 1 in, 7 out]
          }
          event "Tab Control": Value Change {
            n280 = event-data() -> ("NewVal"=w632:T5)  [unwired: 1 out]
            n281 = case shown="\"Templates\"" w632 {
              tunnel: w631 -> [w636 w639 w641 w643]
              tunnel: [w635 w638 w642 w643] -> w630
              frame "Templates" {
                n282 = property on="Filter templates by keyword" class="Str"(error in=w636, "Key Focus"=TRUE) -> (error out=w635:errorcluster)  [unwired: 1 in, 1 out]
              }
              frame "Glyphs" {
                n283 = property on="Filter glyphs by keyword" class="Str"(error in=w639, "Key Focus"=TRUE) -> (error out=w638:errorcluster)  [unwired: 1 in, 1 out]
              }
              frame "Icon Text" {
                n284 = property on="Line 1 text" class="Str"(error in=w641, "Key Focus"=TRUE) -> (error out=w642:errorcluster)  [unwired: 1 in, 1 out]
              }
              frame "Layers", Default {
              }
            }
            n285 = call "NIIE_Finalize Text.vi"("Error"=w630, "Data"=w627) -> ("Error Out"=w633:errorcluster, "Data Out"=w626:T28)  [unwired: 8 out]
            n286 = call "NIIE_Finalize Movement.vi"("Error"=w633, "Data"=w626) -> ("Error Out"=w625:errorcluster, "Data Out"=w623:T28)  [unwired: 1 in, 7 out]
            n287 = call "NIIE_Escape.vi"("Error"=w625, "Data"=w623) -> ("Error Out"=w624:errorcluster, "Data Out"=w622:T28)  [unwired: 1 in, 7 out]
            n288 = call "NIIE_Reset layer template selection.vi"("Error"=w624, "Data"=w622) -> ("Error Out"=w629:errorcluster, "Data Out"=w621:T28)  [unwired: 1 in, 7 out]
          }
          event Mouse Down {
            n289 = event-data() -> ()  [unwired: 2 out]
            n290 = call "NIIE_Finalize Text.vi"("Error"=w650, "Data"=w649) -> ("Error Out"=w651:errorcluster, "Data Out"=w648:T28)  [unwired: 8 out]
            n291 = call "NIIE_Finalize Movement.vi"("Error"=w651, "Data"=w648) -> ("Error Out"=w647:errorcluster, "Data Out"=w645:T28)  [unwired: 1 in, 7 out]
            n292 = call "NIIE_Escape.vi"("Error"=w647, "Data"=w645) -> ("Error Out"=w646:errorcluster, "Data Out"=w644:T28)  [unwired: 1 in, 7 out]
          }
          event Mouse Down {
            n293 = event-data() -> ("Button"=w655:u16)  [unwired: 1 out]
            n294 = case shown="1" w655 {
              tunnel: w657 -> [w659 w663]
              tunnel: [w659 w662] -> w656
              tunnel: w654 -> [w658 w661]
              tunnel: [w658 w660] -> w653
              frame 0, Default {
              }
              frame 1 {
                # "Left click"
                n295 = call "NIIE_Reset layer template selection.vi"("Error"=w663, "Data"=w661) -> ("Error Out"=w662:errorcluster, "Data Out"=w660:T28)  [unwired: 1 in, 7 out]
              }
            }
          }
          event "Preview", "Preview2", "Terminals": Mouse Leave {
            n296 = event-data() -> ()  [unwired: 2 out]
            n297 = Bundle By Name(cluster=w664, "Support.Mouse inside icon?"=FALSE) -> (w666:T28)
          }
          event Mouse Down {
            n298 = event-data() -> ("CtlRef"=w672:refnum<vi>)  [unwired: 1 out]
            n299 = property class="CmbBox (strict)"(reference=w672, error in=w671, "Text.Selection Start"=u32 0 ("Text.Selection:Start"), "Text.Selection End"=u32 1000 ("Text.Selection:End")) -> (error out=w670:errorcluster)  [unwired: 1 out]
          }
          event Value Change {
            n300 = event-data() -> ()  [unwired: 2 out]
            n301 = control-ref of="This VI"() -> (w684:refnum<vi>)
            n302 = call "NIIE_Defer_FP_Updates.vi"("Defer Panel Updates"=TRUE, "error in (no error)"=w683, "lv_icon.vi in"=w684) -> ("error out"=w681:errorcluster, "lv icon.vi out"=w680:refnum<vi>)  [unwired: 7 out]
            n303 = call "NIIE_Add new Layer.vi"("Error"=w681, "Data"=w685) -> ("Error Out"=w676:errorcluster, "Data Out"=w678:T28)  [unwired: 8 out]
            n304 = call "NIIE_Layer_View.vi"("Add To Undo?"=TRUE ("Add to Undo?"), "Error"=w676, "Data"=w678) -> ("Error Out"=w675:errorcluster, "Data Out"=w677:T28)  [unwired: 1 in, 6 out]
            n305 = call "NIIE_Defer_FP_Updates.vi"("error in (no error)"=w675, "lv_icon.vi in"=w680) -> ("error out"=w679:errorcluster)  [unwired: 1 in, 8 out]
          }
          event Value Change {
            n306 = event-data() -> ()  [unwired: 2 out]
            n307 = control-ref of="This VI"() -> (w696:refnum<vi>)
            n308 = Unbundle By Name(w702) -> ("Class.Icon"=w701:refnum<class "Icon.lvclass">)
            n309 = call "NIIE_Defer_FP_Updates.vi"("Defer Panel Updates"=TRUE, "error in (no error)"=w695, "lv_icon.vi in"=w696) -> ("error out"=w694:errorcluster, "lv icon.vi out"=w693:refnum<vi>)  [unwired: 7 out]
            n310 = call-dynamic "GET_All User Layers.vi"("error in (no error)"=w694, "Icon.lvclass in"=w701) -> ("error out"=w708:errorcluster, "User Layer"=w704:refnum<class "Layer.lvclass">[], "Icon.lvclass out"=w703:refnum<class "Icon.lvclass">)  [unwired: 7 out]
            n311 = call "NIIE_Delete Selected Layers.vi"("Error"=w708, "All Layers"=w704, "Data"=w702) -> ("Error Out"=w707:errorcluster, "All Layers Out"=w705:refnum<class "Layer.lvclass">[], "Data Out"=w699:T28)
            n312 = call-dynamic "SET_UserLayers.vi"("error in (no error)"=w707, "Layers"=w705, "Icon.lvclass in"=w703) -> ("error out"=w706:errorcluster, "Icon.lvclass out"=w700:refnum<class "Icon.lvclass">)  [unwired: 7 in]
            n313 = Bundle By Name(cluster=w699, "Class.Icon"=w700) -> (w698:T28)
            n314 = call "NIIE_Reset layer template selection.vi"("Error"=w706, "Data"=w698) -> ("Error Out"=w687:errorcluster, "Data Out"=w689:T28)  [unwired: 1 in, 7 out]
            n315 = call "NIIE_Layer_View.vi"("Add To Undo?"=TRUE ("Add to Undo?"), "Error"=w687, "Data"=w689) -> ("Error Out"=w686:errorcluster, "Data Out"=w688:T28)  [unwired: 2 in, 5 out]
            n316 = call "NIIE_Defer_FP_Updates.vi"("error in (no error)"=w686, "lv_icon.vi in"=w693) -> ("error out"=w692:errorcluster)  [unwired: 1 in, 8 out]
          }
          event Panel Close? {
            w710 = FALSE ("Yes")
            n317 = event-data() -> ()  [unwired: 2 out]
            n318 = event-data("Discard?"=TRUE) -> ()  [unwired: 1 in, 1 out]
          }
          event Mouse Up {
            n319 = event-data() -> ()  [unwired: 2 out]
            n320 = Unbundle By Name(w721) -> ("Support.Action"=w719:T32, "Support.Mouse inside icon?"=w724:bool, "Support.Mouse Move Coords"=w720:T31)
            n321 = case shown="False" w724 {
              tunnel: w722 -> [w728 w739]
              tunnel: [w726 w739] -> w717
              tunnel: [w729 w738] -> w715
              tunnel: w721 -> [w730 w738]
              tunnel: w720 -> [w727 _]
              tunnel: w719 -> [w725 _]
              frame False {
                n322 = case shown="\"Move Selection\", \"Tool\"" w725 {
                  tunnel: w730 -> [w732 w737]
                  tunnel: [w732 w736] -> w729
                  tunnel: w728 -> [w731 w735]
                  tunnel: w727 -> [_ w734]
                  tunnel: [w731 w733] -> w726
                  frame "Default", Default {
                  }
                  frame "Move Selection", "Tool" {
                    n323 = call "NIIE_PictureControl_MouseUp.vi"("Error"=w735, "Coords"=w734, "Data"=w737) -> ("Error Out"=w733:errorcluster, "Data Out"=w736:T28)  [unwired: 4 in, 3 out]
                  }
                }
              }
              frame True {
              }
            }
            n324 = call "NIIE_Undo_Add Data to History.vi"("Check Special Fields? (F)"=TRUE ("Check special fields? (F)"), "Add To Undo?"=TRUE ("Add to Undo?"), "Error"=w717, "Data"=w715) -> ("Error Out"=w716:errorcluster, "Data Out"=w714:T28)  [unwired: 6 out]
          }
          event "Glyphs []": Mouse Down {
            n325 = event-data() -> ("Button"=w748:u16, "Mods.Double Click"=w749:bool, "CtlRef"=w751:refnum<vi>, "Coords"=w752:T31)  [unwired: 1 out]
            n326 = case shown="1" w748 {
              tunnel: w752 -> [_ w761]
              tunnel: w751 -> [_ w760]
              tunnel: [w754 w759] -> w745
              tunnel: w750 -> [w754 w758]
              tunnel: w749 -> [_ w757]
              tunnel: w743 -> [w753 w756]
              tunnel: [w753 w755] -> w741
              frame 0, Default {
              }
              frame 1 {
                # "Left Click"
                n327 = call "NIIE_Mouse Down_Glyphs.vi"("Double Click"=w757, "Coords"=w761, "Error"=w758, "CtlRef"=w760, "Data"=w756) -> ("Error Out"=w759:errorcluster, "Data Out"=w755:T28)  [unwired: 1 in, 4 out]
              }
            }
            n328 = call "NIIE_Reset layer template selection.vi"("Error"=w745, "Data"=w741) -> ("Error Out"=w744:errorcluster, "Data Out"=w742:T28)  [unwired: 1 in, 7 out]
            n329 = call "NIIE_Update glyph path string.vi"("Error"=w744, "Data"=w742) -> ("Error Out"=w746:errorcluster, "Data Out"=w740:T28)  [unwired: 1 in, 7 out]
          }
          event Mouse Down {
            n330 = event-data() -> ()  [unwired: 2 out]
            n331 = call "NIIE_Escape.vi"("Error"=w763, "Data"=w765) -> ("Error Out"=w762:errorcluster, "Data Out"=w764:T28)  [unwired: 1 in, 7 out]
          }
          event "Glyphs", "Templates": Item Close; "Glyphs", "Templates": event #0x1e {
            n332 = event-data() -> ("CtlRef"=w766:refnum<vi>)  [unwired: 1 out]
            n333 = call "NIIE_Tree_DealWithScrollbars.vi"("Error"=w768, "Tree"=w766) -> ("Error Out"=w767:errorcluster)  [unwired: 9 in]
          }
          event Value Change {
            n334 = event-data() -> ()  [unwired: 2 out]
            n335 = Unbundle By Name(w772) -> ("Ref.GlyphLoadAnimation"=w770:refnum<vi>, "Ref.refreshGlyphs"=w771:refnum<vi>)
            n336 = call "NIIE_Launch Dynamically Load Graphics.vi"("User events"=w773, "Path"=Pathes."Glyphs", "error in (no error)"=w775, "button ref"=w771, "animatedDecoration ref"=w770) -> ("error out"=w774:errorcluster)  [unwired: 1 in, 5 out]
          }
          event Value Change {
            n337 = event-data() -> ()  [unwired: 2 out]
            n338 = Unbundle By Name(w779) -> ("Ref.TemplateLoadAnimation"=w777:refnum<vi>, "Ref.refreshTemplates"=w778:refnum<vi>)
            n339 = call "NIIE_Launch Dynamically Load Graphics.vi"("User events"=w780, "Path"=Pathes."Icon Templates", "error in (no error)"=w782, "button ref"=w778, "animatedDecoration ref"=w777) -> ("error out"=w781:errorcluster)  [unwired: 1 in, 5 out]
          }
        }
        n340 = case shown="True" w147 {
          tunnel: [_ w788] -> w151
          tunnel: w150 -> [w785 w791]
          tunnel: [w785 w790] -> w149
          tunnel: "Tools" -> [_ w789]
          tunnel: w143 -> [w784 w787]
          tunnel: [w784 w786] -> w142
          frame False {
          }
          frame True {
            n341 = call "NIIE_DrawIcon.vi"("Tools"=w789, "Error"=w791, "Data"=w787) -> ("Error Out"=w790:errorcluster, "Icon Out"=w788:picture, "Data Out"=w786:T28, "RGB Out"=→"RGB":string, "XYL Out"=→"XYZ":string)  [unwired: 2 in, 2 out]
            "Icon" <- w788
            "Preview" <- w788
          }
        }
        n342 = Unbundle By Name(w150) -> ("status"=w156:bool)
        n343 = Or(x=w156, y=w155) -> (x .or. y?=w154:bool)
      }
      n344 = call "NIIE_Extract LV Icon Data.vi"("Error"=w119, "LabVIEW Icon In (original)"=w117, "Data"=w121) -> ("Error Out"=w118:errorcluster, "LabVIEW Icon Out"=w120:string, "Data Out"=w116:T28)  [unwired: 6 in]
      n345 = call "Get Image Data.vi"("Depth (24)"=24 ("depth (24)"), "Pic"=w136) -> ("Image Data Out"=w124:T4)  [unwired: 1 in, 8 out]
      n346 = call "Get Image Data.vi"("Depth (24)"=1 ("depth"), "Pic"=w136) -> ("Image Data Out"=w134:T4)  [unwired: 1 in, 8 out]
      n347 = call "NIIE_SetCursor.vi"("Radio Buttons"=Cluster_Button_Draw_Tools."Select", "Data"=w116) -> ("Data Out"=w115:T28)  [unwired: 8 in, 1 out]
      n348 = Unbundle By Name(w118) -> ("code"=w137:i32)
      n349 = flat-sequence {
        tunnel: w140 -> [w808]
        tunnel: w138 -> [w805]
        tunnel: w118 -> [w804]
        tunnel: w128 -> [w802]
        tunnel: w115 -> [w798]
        tunnel: w112 -> [w796]
        tunnel: [w796] -> w111
        tunnel: [w795] -> w110
        tunnel: [w794] -> w109
        tunnel: w108 -> [w794]
        tunnel: w111 -> [w813]
        tunnel: w110 -> [w812]
        tunnel: w109 -> [w810]
        frame #0 {
          n350 = Unbundle By Name(w802) -> ("Global stop?"=w801:refnum<user-event>, "Templates"=w800:refnum<user-event>, "Glyphs"=w799:refnum<user-event>)
          n351 = Unbundle(w808) -> ("Events Out"=w807:refnum<event-registration>)
          n352 = call "NIIE_Write INI Tokens and VI Tags.vi"("Error"=w804, "Data"=w798) -> ("Error Out"=w797:errorcluster)  [unwired: 1 in, 8 out]
          n353 = Unregister For Events(event registration refnum=w807) -> ()  [unwired: 1 in, 1 out]
          n354 = flat-sequence {
            tunnel: w797 -> [_]
            tunnel: [w809] -> w795
            frame #0 {
              n355 = call "Caller VI_Call Keep IE in Memory.vi"() -> ()  [unwired: 1 out]
            }
            frame #1 {
              n356 = property class="VI"() -> ("Front Panel.WinBounds"=w809:T38)  [unwired: 2 in, 2 out]
            }
          }
          n357 = Release Notifier(notifier=w805, force destroy? (F)=TRUE) -> ()  [unwired: 1 in, 3 out]
          n358 = Generate User Event(user event=w801, event data cluster=TRUE) -> ()  [unwired: 2 in, 2 out]
          n359 = Destroy User Event(user event=w800) -> ()  [unwired: 1 in, 1 out]
          n360 = Destroy User Event(user event=w799) -> ()  [unwired: 1 in, 1 out]
        }
        frame #1 {
          n361 = Equal?(x=w812, y=w813) -> (x = y?=w811:bool)
          n362 = case shown="False" w811 {
            tunnel: w812 -> [w821 _]
            tunnel: w810 -> [w814 _]
            frame False {
              # "Bounds changed...write new bounds\nto INI file"
              n363 = Unbundle(w821) -> ("Left"=w820:i16, "Top"=w819:i16, "Right"=w818:i16, "Bottom"=w817:i16)
              n364 = Format Into String(format string="%d,%d,%d,%d", w820, w819, w818, w817) -> (resulting string=w815:string)  [unwired: 2 in, 1 out]
              n365 = call-by-ref "?"("value"=w815, "key"=w814) -> ()  [unwired: 3 in, 7 out]
            }
            frame True {
              # "Bounds didn't change while window was\nopen...don't do anything"
            }
          }
        }
        frame #2 {
          n366 = invoke class="VI" method="FP.Close"() -> ()  [unwired: 3 in, 3 out]
        }
      }
      n367 = call-dynamic "GET_Notifier.vi"("error in (no error)"=w122, "Ants.lvclass in"=w126) -> ("error out"=w132:errorcluster, "Notifier"=w138:refnum<notifier>, "Ants.lvclass out"=w133:refnum<class "Ants.lvclass">)  [unwired: 7 out]
      n368 = call "RunningAnts.vi"("error in (no error)"=w132, "Ants in"=w133) -> ()  [unwired: 10 out]
    }
    frame Error {
      n369 = Unbundle By Name(w823) -> ("code"=w824:i32)
      n370 = call <vilib>:"Simple Error Handler.vi"("error in (no error)"=w823) -> ()  [unwired: 4 in, 5 out]
    }
  }
  "BW Icon Out" <- w55
  "Error Code Out" <- w60
  "Color Icon Out" <- w36
  "LabVIEW Icon out" <- w29
